vi "Multi_Run_Prog.vi"(0 "Command filename":path, 1 "Setup mode":T9(ring)) -> ()   [LabVIEW 2011]
uses:
  Anemometry Sub Vis/Gen Trav/Traverse_cluster.ctl
  Anemometry Sub Vis/Gen Trav/Spacing.ctl
  Anemometry Sub Vis/Controls/Multi_run_mode.ctl
  Anemometry Sub Vis/Gen Trav/Route mapping/Route_Display_Mode.ctl
  Anemometry Sub Vis/Controls/User_Specific_mode.ctl
  Anemometry Sub Vis/Controls/Multi_Run_Case.ctl
  Anemometry Sub Vis/Gen Trav/Multi_Run_Status.ctl
  Anemometry Sub Vis/Controls/Tunnel_Coordinates.ctl
  Anemometry Sub Vis/Controls/Post_Process.ctl
  ADAM Client/Sub VIs/ADAM Controls/Traverse_Level_State.ctl
  ADAM Client/Sub VIs/ADAM Controls/Tunnel_speed_mode.ctl
  Anemometry Sub Vis/Controls/Overhead.ctl
  ADAM Client/Sub VIs/ADAM Controls/Remember_value_mode.ctl
  Anemometry Sub Vis/Gen Trav/Trav_mode.ctl
  ADAM Client/Sub VIs/ADAM Controls/Client_Source_Status.ctl
  ADAM Client/Sub VIs/ADAM Controls/Update_scan_value.ctl
  Anemometry Sub Vis/File/Setup_Filetype.ctl
  Anemometry Sub Vis/Globals/Meas_global.vi
  Anemometry Sub Vis/Globals/Trav_pos_global.vi
  Anemometry Sub Vis/Globals/Preference_global.vi
  Anemometry Sub Vis/Gen Trav/Route mapping/Route_mapping_global.vi
  ADAM Serial/Instrument drivers/Traverses/~subVIs/DriveConfigGlobal.vi
  Anemometry Sub Vis/Globals/Extra_Commands_Global.vi
  Anemometry Sub Vis/Globals/LDA_meas_global_2.vi
  Anemometry Sub Vis/Globals/LDA_meas_global_1.vi
panel:
  out "Last Row Run":i32
  in  "Stop after Repeats":bool
  in  "Jump Bad Positions":bool
  in  "Work in Tunnel Coordinates?":T1
  out "Current Overhead Factor":dbl format="%.3f"
  out "Estimated Completion time":string
  out "Max Tunnel Speed":dbl format="%.2f"
  out "Pause message":string
  in  "Pause":bool
  out "Non Starter":bool
  out "No of Rows":i32
  out "Status":T2
  in  "Synchronization Start No":i32=1 min=1 max=100
  out "Multi Run Case":T3
  out "Simulate/Run":T4
  in  "Display Mode":T5=enum."Display View on Crash"
  in  "stop":bool
  out "Currently on Row":i32
  in  "Table":T6[](array[typedef]) {"Row Duration (mins)" format="%#.1f"; "Row No" min=0; "Trace Gas Concentration (%)" min=0.0 format="%#.2f"; "Emission Rate (l/min)" format="%#.2f"; "Tunnel Speed" format="%#.2f"; "Start X" format="%#.2f"; "Start Y" format="%#.2f"; "Start Z" format="%#.2f"; "End X" format="%#.2f"; "End Y" format="%#.2f"; "End Z" format="%#.2f"; "Averaging time (min)" min=0.0 format="%#.2f"}
  # "X           Y            Z"
  # "Start"
  # "End"
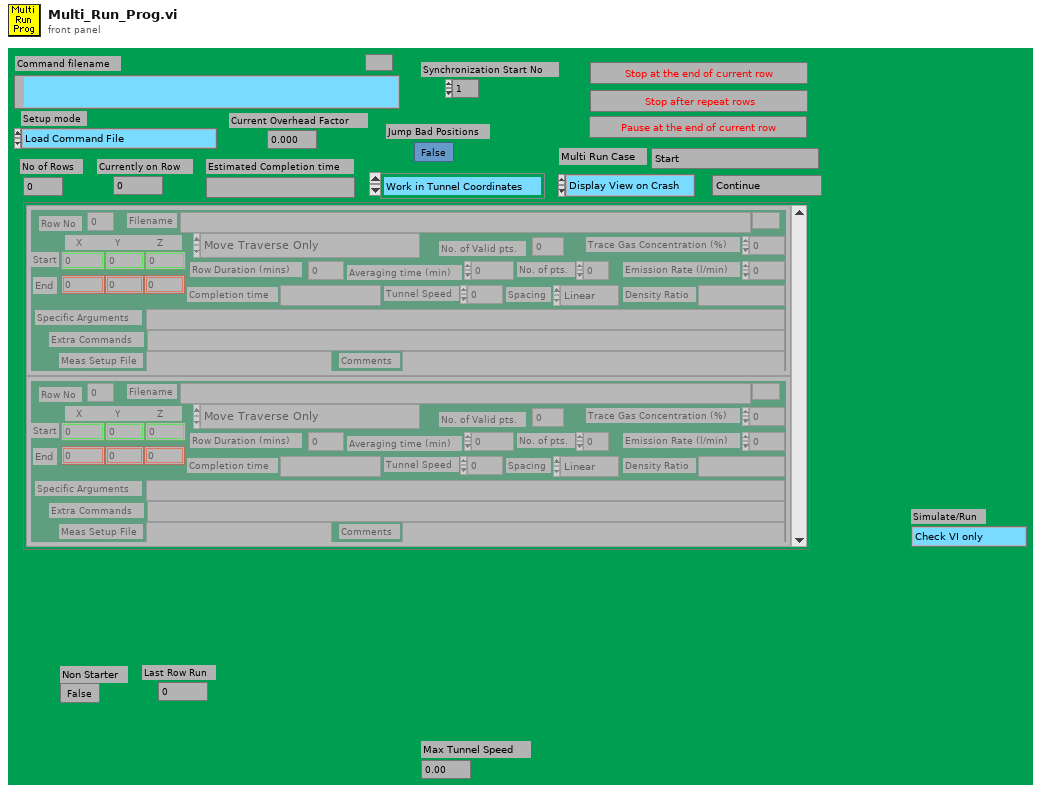
[diagram p1: front panel]
types:
  T1 = typedef "Tunnel_Coordinates.ctl" = enum16{"Work in Tunnel Coordinates", "Work in Model Coordinates"}
  T2 = typedef "Multi_Run_Status.ctl" = enum16{"Continue", "Jump to Next Point", "Jump to Next Row", "Jump To Fall Back", "Terminate Run"}
  T3 = typedef "Multi_Run_Case.ctl" = enum16{"Start", "Load Setup From File", "Has file been edited in Excel?", "Check Max Tunnel Speed", "Pre Check Row", "Check Rows", "Remove blank end rows", "Do results files already exist?", "FFID Bkgnd Measurements?", "First Save Setup file", "Setup Route checking", "Initialise Measurement Prog", "Input Current Position", "Experimental setup control", "Check source flowrates", "Setup for running mode", "Skip Blank Rows", "Which row to execute next", "Evaluate IF Statement", "Perform Measurement Setup", "Set Measurement Conditions", "Execute Row", "Calculate Row TIme", "Update time estimate", "Pause Multi Run Program", "Do Another Row?", "Find Next Fall Back Row", "Shut down source etc", "Email results to users", "Save run efficiency", "Remove Skipped Commands", "Show jumped positions", "Save Setup to File", "End"}
  T4 = typedef "User_Specific_mode.ctl" = enum16{"Check VI only", "Run VI"}
  T5 = typedef "Route_Display_Mode.ctl" = enum16{"Display View Always", "Display View on Crash"}
  T6 = typedef "Traverse_cluster.ctl" = cluster{"Start X":dbl, "Start Y":dbl, "Start Z":dbl, "End X":dbl, "End Y":dbl, "End Z":dbl, "No. of pts.":i32, "Spacing":T7, "Filename":path, "Tunnel Speed":dbl, "Averaging time (min)":dbl, "Extra Commands":string, "Specific Arguments":string, "Emission Rate (l/min)":dbl, "Trace Gas Concentration (%)":dbl, "Density Ratio":string, "Comments":string, "Row No":i32, "Row Type Selector":T8, "Completion time":string, "Row Duration (mins)":dbl, "No. of Valid pts.":i32, "Meas Setup File":string}
  T7 = typedef "Spacing.ctl" = enum16{"Linear", "Log", "Gauss", "Specified", "N/A"}
  T8 = typedef "Multi_run_mode.ctl" = enum16{"Move Traverse Only", "Set Tunnel Speed Only", "Set Source Only", "Set Measurement Conditions", "Single Measurement", "Vertical Profile", "Lateral Profile", "Longitudinal Profile", "Explore Volume", "Multi-Axis Profile", "Auto Calibrate", "Meas Fast FID Bkgnd", "Check Beam Power", "Scanning Valve Measurement", "Run VI Named:", "Set ADAM Ch", "Wait (minutes)", "Send Message", "Synchronize With:", "Fall Back to this Row", "Turn Off Row Repeating", "Blank Row"}
  T9 = enum16{"Load Command File", "Save Command File", "Check Multi Run Prog", "Check Multi Run Prog With Live Moves", "Run Multi Run Prog"}
  T10 = typedef "Post_Process.ctl" = enum16{"Take New Data", "Post Process Raw Data File"}
  T11 = typedef "Traverse_Level_State.ctl" = enum16{"Running", "Complete"}
  T12 = enum32{"existing file", "new file", "new or existing file", "existing dir", "new dir", "new or existing dir", "existing file (use LLBs)", "new file (use LLBs)", "new or existing file (use LLBs)", "new or existing file or directory (use LLBs)"}
  T13 = typedef "Tunnel_speed_mode.ctl" = enum16{"Set Speed", "Set Speed then wait", "Is tunnel speed allowable?"}
  T14 = enum16{"All Channel Names", "Valid Channel Names"}
  T15 = typedef "Overhead.ctl" = enum16{"Update total times", "Read Current Overhead", "Re Scale totals to 3 hrs", "Initialise totals to 3hr"}
  T16 = typedef "Remember_value_mode.ctl" = enum16{"Read only", "Read and Write"}
  T17 = typedef "Trav_mode.ctl" = enum16{"Move traverse", "Read traverse position", "Teach Position"}
  T18 = typedef "Client_Source_Status.ctl" = enum16{"Not Using", "Using", "Must Have"}
  T19 = typedef "Update_scan_value.ctl" = cluster{"Channel Name":string, "New Value":dbl}
  T20 = typedef "Setup_Filetype.ctl" = enum16{"Measurement Setups", "Calibration Setups", "General", "Results File Plotter Setups", "Speed Calib Tweaks"}
  T21 = typedef "AxisConfigCluster.ctl" = cluster{"Channel Properties":T22, "Static Drive Configuration":T23}
  T22 = typedef "DriveProperties.ctl" = cluster{"Channel Name":string, "Vel. Default":dbl, "Acc. Default":dbl, "Vel. Max":dbl, "Vel. Min":dbl, "Acc. Max":dbl, "Acc. Min":dbl, "Pulses/unit":dbl, "Address":u8, "Pulse Offset":i32, "Pos Tolerance":dbl, "Pulses/rev":dbl, "Backlash/Eng units":dbl, "Current Pos":dbl, "Ch Status":enum16{"Active", "Offline", "Simulate"}, "Port Name":string, "Axis Transform mode":string, "Metadata Ch Name":string, "Type":string}
  T23 = typedef "DriveStaticConfig.ctl" = cluster{"Correction Gain % (CG)":u16, "Dead Band (DB)":i32, "Dead Band Window (DW)":i32, "Encoder Resolution (ER)":i32, "Step Mode  (FSB)":u16, "Position Maintenance (FSC)":u16, "Stop on Stall (FSD)":u16, "Activate OP1 on stall (FSE)":u16, "Stop on Trigger 3 (FSF)":u16, "OP2 in Deadband (FSG)":u16, "Stall Detect (FSH)":u16, "Limit Disable (LD)":u16, "Motor Resolution (MR)":enum16{"200", "400", "1000", "2000", "4000", "5000", "10000", "12800", "18000", "20000", "21600", "25000", "25400", "25600", "36000", "50000", "278528", "425984", "507904", "614400", "655360", "819200", "1024000"}, "Limit Switch Sense (OSA)":u16, "Home Position (OSB)":u16, "Home Switch Sense (OSC)":u16, "Encoder Z for Home (OSD)":u16, "Reference edge of Home (OSH)":u16, "RS232 Echo Control (SSA)":u16, "Buffer at Limit (SSG)":u16, "Buffer at Stop (SSH)":u16, "Indexer Mode  (FSA)":u16, "Type":string, "ConfigString":string, "De Power Motor":enum16{"TRUE", "FALSE"}}
  T24 = typedef "Status_Cluster.ctl" = cluster{"Status":T2, "Error Type":string, "Error Description":string}
  T25 = typedef "BSA_info_Cluster.ctl" = cluster{"GPIB Address":string, "No of Check Bytes":i32, "Extra Info":string, "COLOUR":u32, "Wavelength (nm)":dbl}
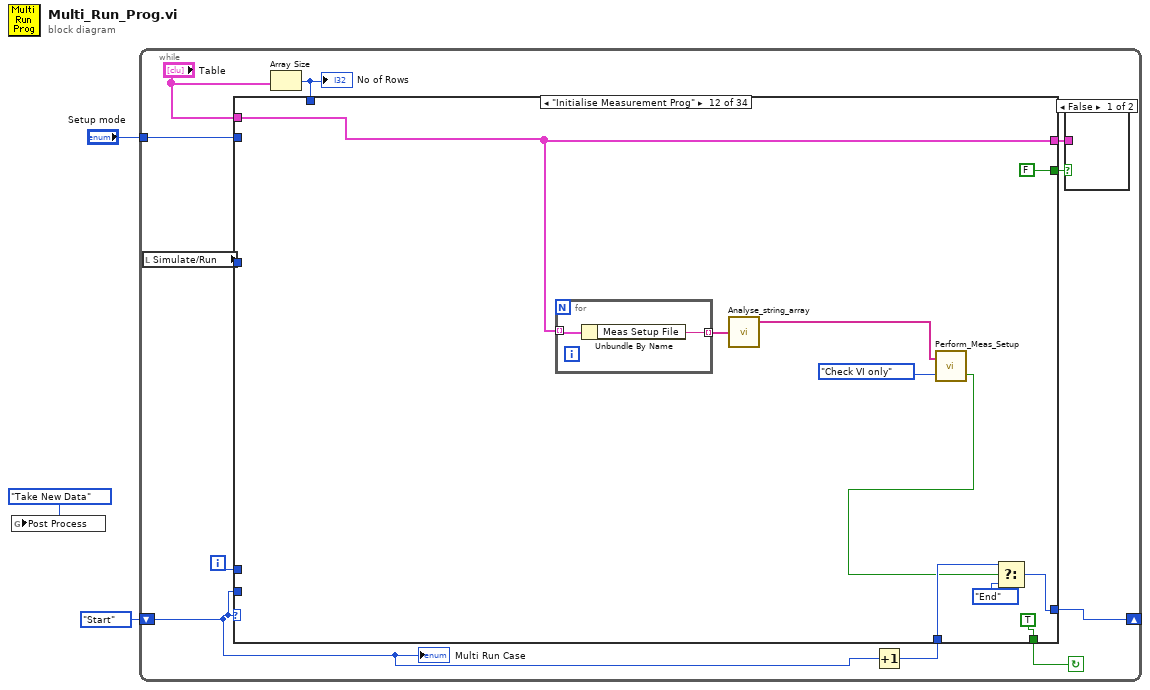
[diagram p0: block diagram]
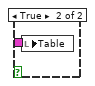
[diagram p2: hidden frame]
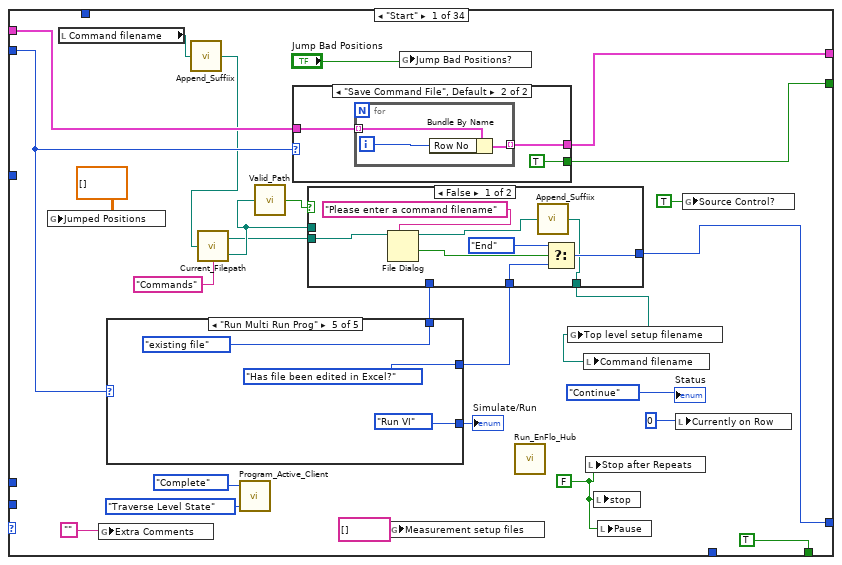
[diagram p3: hidden frame]
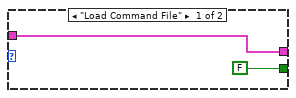
[diagram p4: hidden frame]
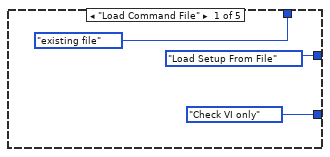
[diagram p6: hidden frame]
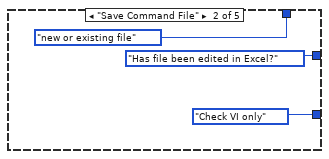
[diagram p7: hidden frame]
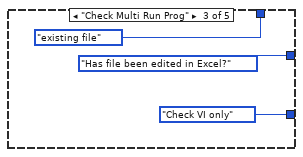
[diagram p8: hidden frame]
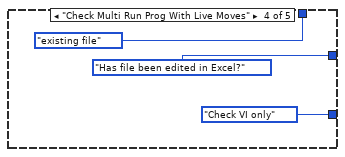
[diagram p9: hidden frame]
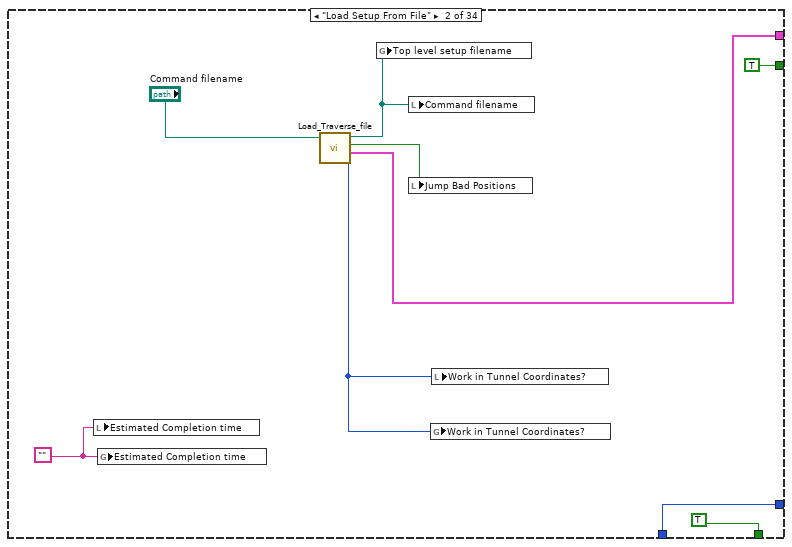
[diagram p10: hidden frame]
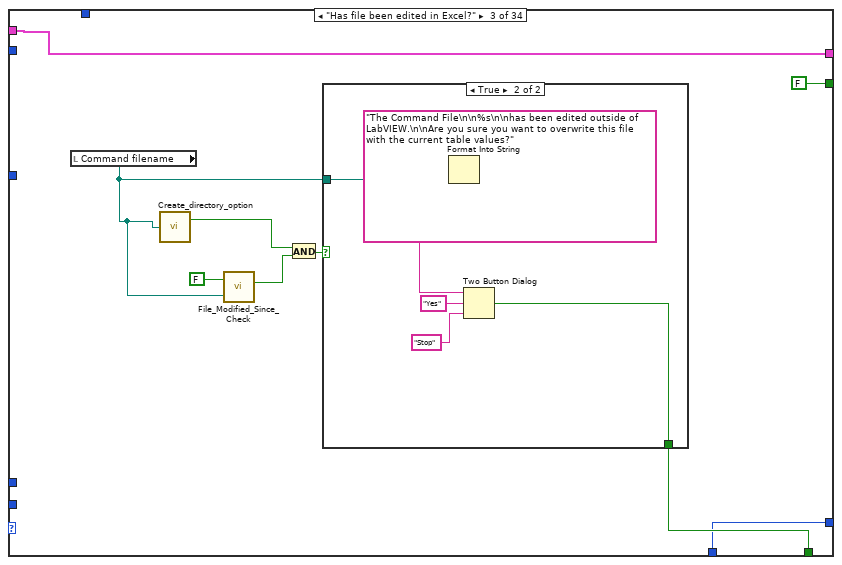
[diagram p11: hidden frame]
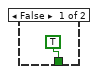
[diagram p12: hidden frame]
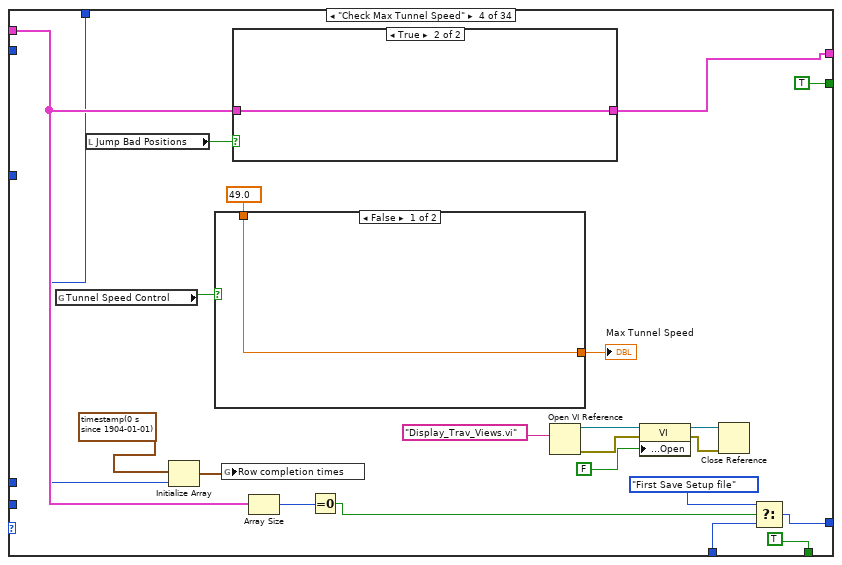
[diagram p13: hidden frame]
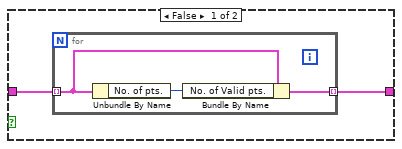
[diagram p14: hidden frame]
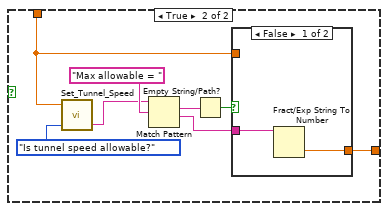
[diagram p15: hidden frame]
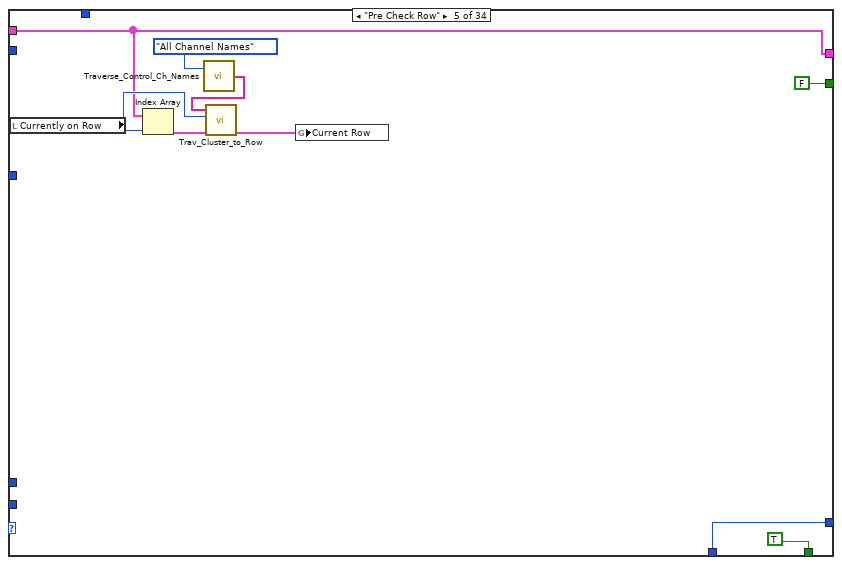
[diagram p17: hidden frame]
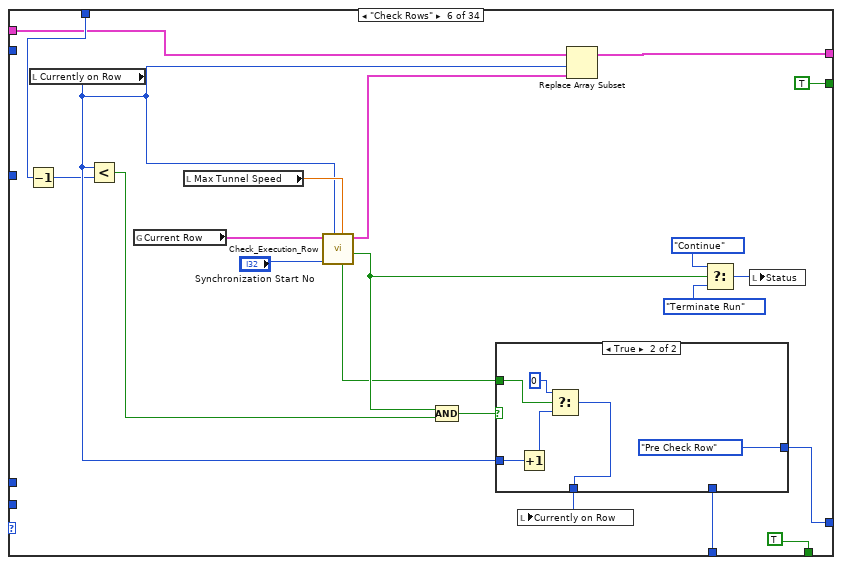
[diagram p18: hidden frame]
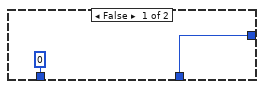
[diagram p19: hidden frame]
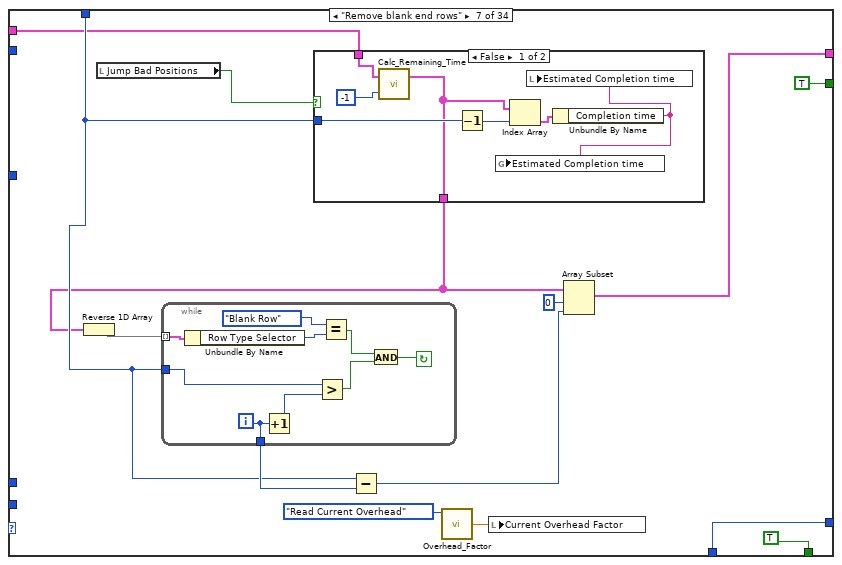
[diagram p20: hidden frame]
diagram:
  n1 = global write "Meas_global.vi" "Post Process"(Post_Process."Take New Data" ("Post Process")) -> ()
  n2 = while {
    shift-left: Multi_Run_Case."Start" ("Multi Run Case") -> [w10]
    shift-right: [w6] -> _
    tunnel: "Setup mode" -> [w13]
    i -> [w11]
    stop <- w14 continue-if-true
    n3 = local read "Simulate/Run"() -> (w7:T4)
    n4 = Array Size(array="Table") -> (size(s)=w5:i32)
    "No of Rows" <- w5
    n5 = Increment(x=w10) -> (x+1=w12:T3)
    n6 = case shown="\"Initialise Measurement Prog\"" w10 {
      tunnel: [TRUE TRUE w87 TRUE TRUE TRUE TRUE TRUE TRUE TRUE TRUE ("Continue?") TRUE ("Continue?") TRUE TRUE TRUE w506 TRUE ("Continue?") TRUE ("Continue?") TRUE TRUE ("Continue?") TRUE TRUE TRUE TRUE TRUE TRUE TRUE TRUE TRUE TRUE TRUE TRUE TRUE FALSE] -> w14
      tunnel: w13 -> [w26 _ _ _ _ _ _ _ _ w395 _ _ _ _ _ _ _ _ _ _ _ _ _ _ _ _ _ _ _ _ _ _ w1220 _]
      tunnel: "Table" -> [w39 _ w84 w114 w142 w154 w179 w210 w368 w397 w419 w472 w477 w483 w493 w509 w561 w605 w721 w772 w784 w875 w911 w943 w984 w1026 w1061 w1091 w1120 w1165 w1170 w1179 w1241 w1304]
      tunnel: w7 -> [_ _ _ _ _ _ _ w209 _ _ _ _ _ w487 w492 w508 _ w603 w718 w769 w782 w874 w909 w940 _ w1035 _ w1082 _ _ _ _ w1231 _]
      tunnel: w10 -> [_ _ _ _ _ _ _ _ _ _ _ _ _ _ _ _ _ _ _ _ _ _ _ _ _ _ _ _ _ _ _ _ _ _]
      tunnel: w12 -> [_ w80 w86 w112 w146 w156 w190 w214 w363 w394 w423 w470 w478 w482 w498 w511 w563 w601 w726 w773 w791 w872 w901 w945 w987 _ _ w1075 w1122 w1167 w1173 w1187 w1239 w1303]
      tunnel: w11 -> [_ _ _ _ _ _ _ _ _ _ _ _ _ _ _ _ _ _ _ _ _ _ _ _ w985 _ _ _ _ _ _ _ _ _]
      tunnel: [w37 w80 w86 w111 w146 w155 w190 w214 w363 w390 w423 w469 w478 w482 w495 w511 w563 w602 w725 w773 w792 w872 w901 w945 w988 w1036 w1058 w1086 w1122 w1167 w1173 w1187 w1239 w1303] -> w6
      tunnel: [w25 TRUE FALSE ("Rows Added ?") TRUE ("Rows Added ?") FALSE TRUE TRUE FALSE FALSE TRUE FALSE FALSE FALSE FALSE FALSE TRUE FALSE ("Rows Added ?") FALSE ("Rows Added ?") FALSE FALSE ("Rows Added ?") FALSE FALSE FALSE TRUE ("Rows Added ?") FALSE FALSE FALSE FALSE FALSE FALSE TRUE TRUE TRUE FALSE] -> w8
      tunnel: w5 -> [_ _ _ w106 _ w160 w181 _ _ _ _ _ _ _ _ _ w564 w604 _ _ _ _ _ w939 _ w1021 _ _ _ _ _ _ _ _]
      tunnel: [w38 w81 w84 w116 w142 w163 w185 w210 w368 w398 w419 w472 w477 w483 w493 w507 w561 w606 w721 w772 w784 w875 w911 w942 w984 w1026 w1061 w1091 w1120 w1165 w1169 w1179 w1240 w1304] -> w4
      frame "Start" {
        w23 = FALSE ("Measurment setup Found?")
        n7 = global write "Trav_pos_global.vi" "Jumped Positions"(dbl[][] [] ("Jumped Positions")) -> ()
        n8 = local read "Command filename"() -> (w29:path)
        n9 = global write "Meas_global.vi" "Extra Comments"("") -> ()
        n10 = case shown="\"Run Multi Run Prog\"" w26 {
          tunnel: [User_Specific_mode."Check VI only" ("Simulate/Run") User_Specific_mode."Check VI only" ("Simulate/Run") User_Specific_mode."Check VI only" ("Simulate/Run") User_Specific_mode."Check VI only" ("Simulate/Run") User_Specific_mode."Run VI" ("Simulate/Run")] -> w40
          tunnel: [Multi_Run_Case."Load Setup From File" ("Multi Run Case") Multi_Run_Case."Has file been edited in Excel?" ("Multi Run Case") Multi_Run_Case."Has file been edited in Excel?" ("Multi Run Case") Multi_Run_Case."Has file been edited in Excel?" ("Multi Run Case") Multi_Run_Case."Has file been edited in Excel?" ("Multi Run Case")] -> w36
          tunnel: [T12."existing file" ("select mode (2)") T12."new or existing file" ("select mode (2)") T12."existing file" ("select mode (2)") T12."existing file" ("select mode (2)") T12."existing file" ("select mode (2)")] -> w24
          frame "Load Command File" {
          }
          frame "Save Command File" {
          }
          frame "Check Multi Run Prog" {
          }
          frame "Check Multi Run Prog With Live Moves" {
          }
          frame "Run Multi Run Prog" {
          }
        }
        "Simulate/Run" <- w40
        n11 = call "Append_Suffiix.vi"("Results file"=w29) -> ("appended path"=w18:path)
        n12 = call "Current_Filepath.vi"("Filename in"=w18, "Data Type"="Commands") -> ("Filename Out"=w17:path, "Directory"=w16:path)
        n13 = call "Program_Active_Client.vi"("Mode"=enum16{"Program Active", "Traverse Level State"}."Traverse Level State", "Traverse level State"=Traverse_Level_State."Complete") -> ()  [unwired: 1 in, 3 out]
        n14 = call "Valid_Path.vi"("Filename"=w17) -> ("Valid Path?"=w27:bool)
        n15 = case shown="\"Save Command File\", Default" w26 {
          tunnel: w39 -> [w43 w46]
          tunnel: [w43 w45] -> w38
          tunnel: [FALSE TRUE] -> w25
          frame "Load Command File" {
          }
          frame "Save Command File", Default {
            n16 = for {
              tunnel: w46 -> [w49] mode=indexing
              tunnel: [w48] -> w45 mode=indexing
              i -> [w47]
              n17 = Bundle By Name(cluster=w49, "Row No"=w47) -> (w48:T6)
            }
          }
        }
        n18 = case shown="False" w27 {
          tunnel: [w55 w59] -> w37
          tunnel: w36 -> [w56 w59]
          tunnel: w17 -> [_ w58]
          tunnel: [w54 w58] -> w28
          tunnel: w24 -> [_ _]
          tunnel: w16 -> [w50 _]
          frame False {
            n19 = File Dialog(7:"Please enter a command filename" ("prompt"), 11:w50) -> (1:w52:bool, 3:w53:path)  [unwired: 1 in, 6 out]
            n20 = call "Append_Suffiix.vi"("Results file"=w53) -> ("appended path"=w54:path)
            n21 = Select(t=Multi_Run_Case."End" ("Multi Run Case"), s=w52, f=w56) -> (s? t:f=w55:T3)
          }
          frame True {
          }
        }
        n22 = global write "Trav_pos_global.vi" "Measurement setup files"(string[] [] ("Measurement setup files")) -> ()
        n23 = global write "Trav_pos_global.vi" "Jump Bad Positions?"("Jump Bad Positions") -> ()
        n24 = call "Run_EnFlo_Hub.vi"() -> ()  [unwired: 8 out]
        n25 = global write "Trav_pos_global.vi" "Top level setup filename"(w28) -> ()
        n26 = local write "Command filename"(w28) -> ()
        n27 = local write "Stop after Repeats"(w23) -> ()
        n28 = local write "stop"(w23) -> ()
        n29 = local write "Pause"(w23) -> ()
        n30 = local write "Currently on Row"(0 ("Currently on Row")) -> ()
        n31 = global write "Trav_pos_global.vi" "Source Control?"(TRUE ("Source Control?")) -> ()
        "Status" <- Multi_Run_Status."Continue" ("Status")
      }
      frame "Load Setup From File" {
        w76 = ""
        n32 = local write "Estimated Completion time"(w76) -> ()
        n33 = global write "Trav_pos_global.vi" "Estimated Completion time"(w76) -> ()
        n34 = call "Load_Traverse_file.vi"("Setup filename"="Command filename") -> ("Setup filename Out"=w78:path, "Jump Bad Positions"=w75:bool, "Table"=w81:T6[], "Work in Tunnel Coordinates?"=w77:T1)  [unwired: 2 out]
        n35 = global write "Trav_pos_global.vi" "Top level setup filename"(w78) -> ()
        n36 = local write "Command filename"(w78) -> ()
        n37 = local write "Jump Bad Positions"(w75) -> ()
        n38 = global write "Trav_pos_global.vi" "Work in Tunnel Coordinates?"(w77) -> ()
        n39 = local write "Work in Tunnel Coordinates?"(w77) -> ()
      }
      frame "Has file been edited in Excel?" {
        n40 = local read "Command filename"() -> (w88:path)
        n41 = call "Create_directory_option.vi"("Filename"=w88) -> ("Path is to existing File"=w91:bool)  [unwired: 1 out]
        n42 = call "File_Modified_Since_Check.vi"("Pathname"=w88, "Just Modified?"=FALSE) -> ("Modified?"=w90:bool)
        n43 = And(x=w91, y=w90) -> (x .and. y?=w92:bool)
        n44 = case shown="True" w92 {
          tunnel: w88 -> [_ w99]
          tunnel: [TRUE ("T button?") w94] -> w87
          frame False {
          }
          frame True {
            n45 = Format Into String(format string="The Command File\n\n%s\n\nhas been edited outside of LabVIEW.\n\nAre you sure you want to overwrite this file  with the current table values?" ("Format String"), w99) -> (resulting string=w97:string)  [unwired: 2 in, 1 out]
            n46 = Two Button Dialog(message=w97, 1:"Stop" ("F button name (\"Cancel\")"), 2:"Yes" ("T button name (\"OK\")")) -> (T button?=w94:bool)
          }
        }
      }
      frame "Check Max Tunnel Speed" {
        n47 = global read "Preference_global.vi" "Tunnel Speed Control"() -> (w117:bool)
        n48 = local read "Jump Bad Positions"() -> (w115:bool)
        n49 = Initialize Array(timestamp(0 s since 1904-01-01) ("seconds since 1Jan1904"), w106) -> (w107:timestamp[])
        n50 = case shown="False" w117 {
          tunnel: 49.0 ("Tunnel Velocity m/s") -> [w128 w129]
          tunnel: [w128 w131] -> w119
          frame False {
          }
          frame True {
            n51 = call "Set_Tunnel_Speed.vi"("Mode"=Tunnel_speed_mode."Is tunnel speed allowable?", "Tunnel Velocity m/s"=w129) -> ("Error String"=w134:string)  [unwired: 1 in, 2 out]
            n52 = Match Pattern(string=w134, regular expression="Max allowable = ") -> (match substring=w133:string, after substring=w130:string)  [unwired: 3 out]
            n53 = Empty String/Path?(string/path=w133) -> (empty?=w132:bool)
            n54 = case shown="False" w132 {
              tunnel: [w137 w139] -> w131
              tunnel: w129 -> [_ w139]
              tunnel: w130 -> [w138 _]
              frame False {
                n55 = Fract/Exp String To Number(string=w138) -> (number=w137:dbl)  [unwired: 4 out]
              }
              frame True {
              }
            }
          }
        }
        "Max Tunnel Speed" <- w119
        n56 = global write "Trav_pos_global.vi" "Row completion times"(w107) -> ()
        n57 = case shown="True" w115 {
          tunnel: w114 -> [w123 w127]
          tunnel: [w122 w127] -> w116
          frame False {
            n58 = for {
              tunnel: w123 -> [w125] mode=indexing
              tunnel: [w124] -> w122 mode=indexing
              n59 = Unbundle By Name(w125) -> ("No. of pts."=w126:i32)
              n60 = Bundle By Name(cluster=w125, "No. of Valid pts."=w126) -> (w124:T6)
            }
          }
          frame True {
          }
        }
        n61 = Array Size(array=w114) -> (size(s)=w113:i32)
        n62 = Equal To 0?(x=w113) -> (x = 0?=w110:bool)
        n63 = Open VI Reference(vi path="Display_Trav_Views.vi" ("VI path")) -> (vi reference=w105:refnum<vi>, error out=w104:errorcluster)  [unwired: 1 in, 4 out]
        n64 = property class="VI"(reference=w105, error in=w104, "Front Panel Window:Open"=FALSE) -> (reference out=w102:refnum<vi>, error out=w101:errorcluster)
        n65 = Close Reference(reference=w102, error in (no error)=w101) -> ()  [unwired: 1 out]
        n66 = Select(t=Multi_Run_Case."First Save Setup file" ("Multi Run Case"), s=w110, f=w112) -> (s? t:f=w111:T3)
      }
      frame "Pre Check Row" {
        n67 = local read "Currently on Row"() -> (w143:i32)
        n68 = Index Array(array=w142, index=w143) -> (element=w144:T6)
        n69 = call "Traverse_Control_Ch_Names.vi"("Mode"=T14."All Channel Names") -> ("Channel names"=w140:string[])  [unwired: 1 in]
        n70 = call "Trav_Cluster_to_Row.vi"("Traverse line in"=w144, "Row Number"=w143, "Channel names"=w140) -> ("Traverse line Out"=w145:T6)  [unwired: 4 out]
        n71 = global write "Trav_pos_global.vi" "Current Row"(w145) -> ()
      }
      frame "Check Rows" {
        n72 = Decrement(x=w160) -> (x-1=w150:i32)
        n73 = local read "Currently on Row"() -> (w151:i32)
        n74 = Less?(x=w151, y=w150) -> (x < y?=w159:bool)
        n75 = global read "Trav_pos_global.vi" "Current Row"() -> (w152:T6)
        n76 = local read "Max Tunnel Speed"() -> (w162:dbl)
        n77 = call "Check_Execution_Row.vi"("Execution Row"=w152, "Synchronization Start No"="Synchronization Start No", "Row Index"=w151, "Max Tunnel Speed"=w162) -> ("Editted Row"=w149:bool, "Execution Row Out"=w153:T6, "Continue?"=w161:bool)  [unwired: 1 in, 3 out]
        n78 = Compound Arithmetic op=AND(w161, w159) -> (w158:bool)
        n79 = case shown="True" w158 {
          tunnel: [0 w173] -> w157
          tunnel: w151 -> [_ w177]
          tunnel: w156 -> [w171 _]
          tunnel: [w171 Multi_Run_Case."Pre Check Row" ("Multi Run Case")] -> w155
          tunnel: w149 -> [_ w175]
          frame False {
          }
          frame True {
            n80 = Increment(x=w177) -> (x+1=w174:i32)
            n81 = Select(t=0, s=w175, f=w174) -> (s? t:f=w173:i32)
          }
        }
        n82 = local write "Currently on Row"(w157) -> ()
        n83 = Replace Array Subset(array=w154, new element=w153, index=w151) -> (w163:T6[])
        n84 = Select(t=Multi_Run_Status."Continue" ("Status"), s=w161, f=Multi_Run_Status."Terminate Run" ("Status")) -> (s? t:f=w167:T2)
        n85 = local write "Status"(w167) -> ()
      }
      frame "Remove blank end rows" {
        n86 = local read "Jump Bad Positions"() -> (w178:bool)
        n87 = case shown="False" w178 {
          tunnel: w181 -> [w196 _]
          tunnel: w179 -> [w195 w199]
          tunnel: [w193 w199] -> w180
          frame False {
            n88 = call "Calc_Remaining_Time.vi"("Currently on Row"=-1 ("Start Index"), "Table In"=w195) -> ("Table Out"=w193:T6[])  [unwired: 1 out]
            n89 = Decrement(x=w196) -> (x-1=w198:i32)
            n90 = Index Array(array=w193, index=w198) -> (element=w197:T6)
            n91 = Unbundle By Name(w197) -> ("Completion time"=w192:string)
            n92 = global write "Trav_pos_global.vi" "Estimated Completion time"(w192) -> ()
            n93 = local write "Estimated Completion time"(w192) -> ()
          }
          frame True {
          }
        }
        n94 = Reverse 1D Array(array=w180) -> (reversed array=w189:T6[])
        n95 = while {
          tunnel: [w200] -> w187
          tunnel: w181 -> [w204]
          tunnel: w189 -> [w208] mode=indexing
          i -> [w200]
          stop <- w201 continue-if-true
          n96 = Unbundle By Name(w208) -> ("Row Type Selector"=w206:T8)
          n97 = Increment(x=w200) -> (x+1=w205:i32)
          n98 = Greater?(x=w204, y=w205) -> (0:w203:bool)
          n99 = Equal?(x=Multi_run_mode."Blank Row" ("Row Type Selector"), y=w206) -> (x = y?=w202:bool)
          n100 = And(x=w202, y=w203) -> (x .and. y?=w201:bool)
        }
        n101 = Subtract(x=w181, y=w187) -> (x-y=w186:i32)
        n102 = call "Overhead_Factor.vi"("Mode"=Overhead."Read Current Overhead") -> ("Current Overhead Factor"=w182:dbl)  [unwired: 3 in]
        n103 = local write "Current Overhead Factor"(w182) -> ()
        n104 = Array Subset(array=w180, index=0 ("Array Index"), length=w186) -> (w185:T6[])
      }
      frame "Do results files already exist?" {
        n105 = for {
          tunnel: w210 -> [w226] mode=indexing
          tunnel: [w224] -> w216 mode=indexing
          shift-right: [w220] -> _
          shift-left: path[] [] -> [w221]
          tunnel: w209 -> [w218]
          n106 = Unbundle By Name(w226) -> ("Specific Arguments"=w217:string, "Emission Rate (l/min)"=w225:dbl, "Row Type Selector"=w223:T8, "Filename"=w222:path)
          n107 = while {
            shift-left: w221 -> [w234]
            shift-right: [w233] -> w220
            tunnel: w222 -> [w235]
            tunnel: w223 -> [w239]
            shift-left: 0 -> [w240]
            shift-right: [w236] -> _
            tunnel: w218 -> [w230]
            shift-right: [w229] -> _
            shift-left: _ -> [w228]
            tunnel: w217 -> [w227]
            stop <- w238 continue-if-true
            n108 = Increment(x=w240) -> (x+1=w237:i32)
            n109 = case shown="0, Default" w240 {
              tunnel: w239 -> [w249 _ _ _ _ _ _ _ _ _ _ _]
              tunnel: [w244 w269 w274 w281 w286 TRUE ("exists?") TRUE ("exists?") FALSE ("exists?") FALSE ("exists?") TRUE ("true") w343 w356] -> w238
              tunnel: w237 -> [w251 w272 w277 w280 w287 w292 w303 w314 w325 w329 w341 _]
              tunnel: [w251 w272 w277 w280 w287 w290 w302 w314 w325 w330 w341 w355] -> w236
              tunnel: [w250 w271 w276 w279 w284 w300 w311 w316 w318 w327 w345 w361] -> w233
              tunnel: w234 -> [w250 w271 w276 w279 w285 w300 w311 w316 w318 w327 w345 w361]
              tunnel: w235 -> [w243 _ _ _ _ _ _ _ _ _ _ _]
              tunnel: 7 -> [_ _ _ _ _ _ _ _ _ w328 _ w355]
              tunnel: 9 -> [_ _ _ _ _ w291 _ _ _ _ _ _]
              tunnel: w230 -> [_ _ _ _ _ _ _ _ _ _ w344 _]
              tunnel: [w242 w268 w273 w278 w283 w288 w301 w312 w317 w326 w342 w354] -> w229
              tunnel: w228 -> [_ w268 w273 w278 w283 w288 w301 w312 w317 w326 w342 w354]
              tunnel: w227 -> [w241 _ _ _ _ _ _ _ _ _ _ _]
              frame 0, Default {
                n110 = case shown="\"Run VI Named:\"" w249 {
                  tunnel: [TRUE w259 FALSE FALSE] -> w246
                  tunnel: w243 -> [w252 w258 w264 w266]
                  tunnel: w241 -> [_ w256 _ _]
                  tunnel: [w252 w258 w264 w266] -> w242
                  frame "Move Traverse Only", Default {
                  }
                  frame "Run VI Named:" {
                    n111 = Match Pattern(string=w256, regular expression=";") -> (before substring=w255:string)  [unwired: 4 out]
                    n112 = call <vilib>:"Trim Whitespace.vi"("string"=w255) -> ("trimmed string"=w254:string)  [unwired: 1 in]
                    n113 = Equal?(x=w254, y="Pressure_Tapped_Cube.vi") -> (x = y?=w260:bool)
                    n114 = Equal?(x=w254, y="Take_Data_on_the_Move.vi") -> (x = y?=w261:bool)
                    n115 = Or(x=w260, y=w261) -> (x .or. y?=w259:bool)
                  }
                  frame "Auto Calibrate" {
                  }
                  frame "Send Message" {
                  }
                }
                n116 = local read "Status"() -> (w247:T2)
                n117 = Not Equal?(x=Multi_Run_Status."Terminate Run" ("Status"), y=w247) -> (x != y?=w245:bool)
                n118 = And(x=w246, y=w245) -> (x .and. y?=w244:bool)
              }
              frame 1 {
                n119 = Not Equal?(x=path "", y=w268) -> (x != y?=w269:bool)
              }
              frame 2 {
                n120 = Not Equal?(x=w273, y=path "") -> (x != y?=w274:bool)
              }
              frame 3 {
                n121 = Search 1D Array(1D array=w279, element=w278) -> (index of element=w282:i32)  [unwired: 1 out]
                n122 = Less Than 0?(x=w282) -> (x < 0?=w281:bool)
              }
              frame 4 {
                n123 = Build Array (concatenate)(w285, w283) -> (w284:path[])
                n124 = call "Does_file_exist_(simple).vi"("Pathname"=w283) -> ("exists?"=w286:bool)
              }
              frame 5 {
                n125 = Path To String(path=w288) -> (string=w299:string)
                n126 = global read "Meas_global.vi" "Start Time of experiment"() -> (w294:dbl)
                n127 = Concatenate Strings(w299, "Append" ("Substring")) -> (w297:string)
                n128 = call "Remember_value.vi"("Mode"=Remember_value_mode."Read only", "Ch name"=w297) -> ("Output Value"=w295:dbl)  [unwired: 1 in]
                n129 = Not Equal?(x=w294, y=w295) -> (x != y?=w293:bool)
                n130 = Select(t=w292, s=w293, f=w291) -> (s? t:f=w290:i32)
              }
              frame 6 {
                n131 = Increment(x=w303) -> (x+1=w304:i32)
                n132 = Format Into String(format string="The results filename \"%s\" already exists.\nDo you wish to append to this file during the run?" ("Format String"), w301) -> (resulting string=w308:string)  [unwired: 2 in, 1 out]
                n133 = Two Button Dialog(message=w308, 1:"Abort Run" ("F button name (\"Cancel\")"), 2:"Append" ("T button name (\"OK\")")) -> (T button?=w305:bool)
                n134 = Select(t=w304, s=w305, f=w303) -> (s? t:f=w302:i32)
              }
              frame 7 {
                n135 = local write "Status"(Multi_Run_Status."Terminate Run" ("Status")) -> ()
              }
              frame 8 {
                n136 = Path To String(path=w317) -> (string=w324:string)
                n137 = Concatenate Strings(w324, "Append" ("Substring")) -> (w322:string)
                n138 = global read "Meas_global.vi" "Start Time of experiment"() -> (w319:dbl)
                n139 = call "Remember_value.vi"("Mode"=Remember_value_mode."Read and Write", "Input Value"=w319, "Ch name"=w322) -> ()  [unwired: 1 out]
              }
              frame 9 {
                n140 = call "Read_File_Simple.vi"("Filename"=w326) -> ("string"=w333:string)  [unwired: 2 in, 7 out]
                n141 = call "Is_it_a_Results_File.vi"("character string"=w333) -> ("Results File?"=w332:bool)  [unwired: 2 out]
                n142 = case shown="True" w332 {
                  tunnel: w326 -> [w336 _]
                  tunnel: [w334 w340] -> w330
                  tunnel: w329 -> [_ w340]
                  tunnel: w328 -> [w334 _]
                  frame False {
                    n143 = Path To String(path=w336) -> (string=w338:string)
                    n144 = Format Into String(format string="The File %s is not in the correct Results file format.\nCheck that it is tab delimited rather than excel format, or choose another file." ("Format String"), w338) -> (resulting string=w335:string)  [unwired: 2 in, 1 out]
                    n145 = One Button Dialog(message=w335, button name ("OK")="Stop") -> ()  [unwired: 1 out]
                  }
                  frame True {
                  }
                }
              }
              frame 10 {
                n146 = case shown="\"Check VI only\", Default" w344 {
                  tunnel: w342 -> [_ w353]
                  tunnel: [FALSE ("exists?") w347] -> w343
                  frame "Check VI only", Default {
                  }
                  frame "Run VI" {
                    n147 = call "Open_File_for_write.vi"("append to file? (new file:F)"=TRUE, "file path"=w353) -> ("error out"=w351:errorcluster, "refnum"=w352:refnum<file>)  [unwired: 1 in, 7 out]
                    n148 = Unbundle By Name(w351) -> ("code"=w350:i32)
                    n149 = Close File(refnum=w352, error in=w351) -> ()  [unwired: 2 out]
                    n150 = Equal?(x=10 ("code"), y=w350) -> (x = y?=w347:bool)
                  }
                }
              }
              frame 11 {
                n151 = Path To String(path=w354) -> (string=w359:string)
                n152 = Format Into String(format string="The File %s is already open in another application." ("Format String"), w359) -> (resulting string=w358:string)  [unwired: 2 in, 1 out]
                n153 = One Button Dialog(message=w358, button name ("OK")="Stop") -> (true=w356:bool)
              }
            }
          }
          n154 = Greater Than 0?(x=w225) -> (x > 0?=w224:bool)
        }
        n155 = Or Array Elements(Boolean array=w216) -> (logical OR=w212:bool)
        n156 = global write "Trav_pos_global.vi" "Source Control?"(w212) -> ()
      }
      frame "FFID Bkgnd Measurements?" {
        n157 = for {
          tunnel: w368 -> [w384] mode=indexing
          tunnel: [w372] -> w367 mode=indexing
          tunnel: [w373] -> w366 mode=indexing
          n158 = Unbundle By Name(w384) -> ("Row Type Selector"=w378:T8, "Specific Arguments"=w380:string)
          n159 = call "Get_array_values_fr_String.vi"("String Value"=w380) -> ("String array"=w381:string[])  [unwired: 1 out]
          n160 = Index Array(array=w381, index=0 ("Index")) -> (element=w377:string)
          n161 = Equal?(x=Multi_run_mode."Auto Calibrate" ("Row Type Selector"), y=w378) -> (x = y?=w374:bool)
          n162 = Equal?(x=w377, y="Concentration") -> (x = y?=w375:bool)
          n163 = Equal?(x=Multi_run_mode."Meas Fast FID Bkgnd" ("Row Type Selector"), y=w378) -> (x = y?=w372:bool)
          n164 = And(x=w374, y=w375) -> (x .and. y?=w373:bool)
        }
        n165 = Or Array Elements(Boolean array=w367) -> (logical OR=w364:bool)
        n166 = Or Array Elements(Boolean array=w366) -> (logical OR=w365:bool)
        n167 = Compound Arithmetic op=AND(invert w364, w365) -> (w362:bool)
        n168 = case shown="True" w362 {
          frame False {
          }
          frame True {
            n169 = One Button Dialog(message="This run automatically calibrates the Fast FID but does not have a Meas Fast FID Bkgnd row" ("format string")) -> ()  [unwired: 2 out]
          }
        }
      }
      frame "First Save Setup file" {
        w385 = -1 ("Currently on Row")
        n170 = case shown="\"Check Multi Run Prog\"" w395 {
          tunnel: [w402 w404 w406 Multi_Run_Case."End" ("Multi Run Case") Multi_Run_Case."End" ("Multi Run Case")] -> w389
          tunnel: w394 -> [w402 w404 w406 _ _]
          tunnel: [w403 w405 w407 w408 w410] -> w388
          frame "Run Multi Run Prog" {
            w403 = FALSE  # Live Traverse Preview?
          }
          frame "Check Multi Run Prog With Live Moves" {
            w405 = TRUE  # Live Traverse Preview?
          }
          frame "Check Multi Run Prog" {
            w407 = FALSE  # Live Traverse Preview?
          }
          frame "Load Command File" {
            w408 = FALSE  # Live Traverse Preview?
          }
          frame "Save Command File" {
            w410 = FALSE  # Live Traverse Preview?
          }
        }
        n171 = local read "Command filename"() -> (w396:path)
        n172 = global write "Trav_pos_global.vi" "Work in Tunnel Coordinates?"("Work in Tunnel Coordinates?") -> ()
        n173 = local write "Currently on Row"(w385) -> ()
        n174 = local write "Last Row Run"(w385) -> ()
        n175 = local read "Jump Bad Positions"() -> (w386:bool)
        n176 = call "Save_Trav_setup.vi"("Work in Tunnel Coordinates?"="Work in Tunnel Coordinates?", "Trav Table"=w397, "Jump Bad Positions"=w386, "Setup filename"=w396) -> ("Trav Table Out"=w398:T6[])  [unwired: 1 out]
        n177 = global write "Meas_global.vi" "Extra Comments"("") -> ()
        n178 = global write "Trav_pos_global.vi" "Live Traverse Preview?"(w388) -> ()
        n179 = local read "Status"() -> (w391:T2)
        n180 = case shown="\"Continue\"" w391 {
          tunnel: [w400 Multi_Run_Case."End" ("Multi Run Case")] -> w390
          tunnel: w389 -> [w400 _]
          frame "Continue" {
          }
          frame "Jump to Next Point", Default {
          }
        }
      }
      frame "Setup Route checking" {
        w414 = string[] []
        n181 = global read "Trav_pos_global.vi" "Work in Tunnel Coordinates?"() -> (w416:T1)
        n182 = for {
          tunnel: w419 -> [w459] mode=indexing
          shift-right: [w450] -> w417
          shift-left: string[] [] -> [w451]
          n183 = Unbundle By Name(w459) -> ("Extra Commands"=w452:string, "Start X"=w456:dbl, "Start Y"=w455:dbl, "Start Z"=w454:dbl)
          n184 = Build Array(w456, w455, w454) -> (w457:dbl[])
          n185 = Not A Number/Path/Refnum?(number/path/refnum=w457) -> (NaN/Path/Refnum?=w458:bool[])
          n186 = Or Array Elements(Boolean array=w458) -> (logical OR=w453:bool)
          n187 = case shown="False" w453 {
            tunnel: w452 -> [w463 _]
            tunnel: w451 -> [w462 w464]
            tunnel: [w461 w464] -> w450
            frame False {
              n188 = call "Which_Trav_Setup.vi"("Extra Command String"=w463) -> ("Traverse Setup"=w460:string)
              n189 = Build Array (concatenate)(w462, w460) -> (w461:string[])
            }
            frame True {
            }
          }
        }
        n190 = call "Analyse_string_array.vi"("String array"=w417) -> ("Unique strings"=w415:string[])  [unwired: 2 out]
        n191 = for {
          tunnel: w415 -> [w429] mode=indexing
          tunnel: w416 -> [w428]
          shift-right: [w427] -> w412
          shift-left: w414 -> [w426]
          shift-right: [w424] -> w413
          shift-left: w414 -> [w425]
          n192 = stacked-sequence {
            tunnel: w429 -> [w433 w438]
            tunnel: w428 -> [w430 _]
            tunnel: [_ w437] -> w427
            tunnel: w426 -> [_ w436]
            tunnel: w425 -> [_ w435]
            tunnel: [_ w434] -> w424
            frame #0 {
              n193 = call "3D_Traverse_move.vi"("Mode"=Trav_mode."Read traverse position", "Work in Tunnel Coordinates"=w430, "Simulate/Run"=User_Specific_mode."Run VI", "Traverse name"=w433) -> ()  [unwired: 5 in, 7 out]
            }
            frame #1 {
              n194 = global read "DriveConfigGlobal.vi" "Configurations"() -> (w439:T21[])
              n195 = for {
                tunnel: w439 -> [w449] mode=indexing
                tunnel: w438 -> [w446]
                shift-right: [w444] -> w437
                shift-left: w436 -> [w445]
                shift-right: [w440] -> w434
                shift-left: w435 -> [w441]
                i -> [w448]
                n196 = Unbundle By Name(w449) -> ("Channel Properties.Metadata Ch Name"=w443:string)
                n197 = Format Into String(format string="%d", initial string=w446, w448) -> (resulting string=w442:string)  [unwired: 1 in, 1 out]
                n198 = Build Array (concatenate)(w445, w443) -> (w444:string[])
                n199 = Build Array (concatenate)(w441, w442) -> (w440:string[])
              }
            }
          }
        }
        n200 = global write "Trav_pos_global.vi" "ADAM Positions Ch names"(w412) -> ()
        n201 = global write "Route_mapping_global.vi" "Display Mode"("Display Mode") -> ()
        n202 = global write "Trav_pos_global.vi" "Route checking Chs"(w413) -> ()
      }
      frame "Initialise Measurement Prog" {
        n203 = for {
          tunnel: w472 -> [w476] mode=indexing
          tunnel: [w475] -> w466 mode=indexing
          n204 = Unbundle By Name(w476) -> ("Meas Setup File"=w475:string)
        }
        n205 = call "Analyse_string_array.vi"("String array"=w466) -> ("Unique strings"=w465:string[])  [unwired: 1 in, 1 out]
        n206 = call "Perform_Meas_Setup.vi"("Simulate/Run"=User_Specific_mode."Check VI only", "String array"=w465) -> ("Continue?"=w467:bool)  [unwired: 1 out]
        n207 = Select(t=w470, s=w467, f=Multi_Run_Case."End" ("Multi Run Case")) -> (s? t:f=w469:T3)
      }
      frame "Input Current Position" {
        n208 = call "Save_ADAM_Table_Locally.vi"() -> ()  [unwired: 12 in]
      }
      frame "Experimental setup control" {
        n209 = global read "Trav_pos_global.vi" "Source Control?"() -> (w484:bool)
        n210 = Equal?(x=w487, y=User_Specific_mode."Run VI" ("Simulate/Run")) -> (x = y?=w486:bool)
        n211 = Or(x=w484, y=w486) -> (x .or. y?=w485:bool)
        n212 = case shown="True" w485 {
          tunnel: w484 -> [_ w491]
          frame False {
          }
          frame True {
            n213 = call "Exp_Setup_Control_remote.vi"("Dispersion?"=w491) -> ()  [unwired: 3 out]
          }
        }
        n214 = global write "Trav_pos_global.vi" "FFID Background"(T6 {"Start X"=nan, "Start Y"=nan, "Start Z"=nan, "End X"=nan, "End Y"=nan, "End Z"=nan, "No. of pts."=0, "Spacing"=enum."Linear", "Filename"=path "", "Tunnel Speed"=nan, "Averaging time (min)"=nan, "Extra Commands"="", "Specific Arguments"="", "Emission Rate (l/min)"=nan, "Trace Gas Concentration (%)"=nan, "Density Ratio"="", "Comments"="", "Row No"=0, "Row Type Selector"=enum."Blank Row", "Completion time"="", "Row Duration (mins)"=nan, "No. of Valid pts."=0, "Meas Setup File"=""} ("FFID Background")) -> ()
      }
      frame "Check source flowrates" {
        n215 = case shown="\"Run VI\"" w492 {
          tunnel: w493 -> [_ w502]
          frame "Check VI only", Default {
            n216 = Get Date/Time In Seconds() -> (seconds since 1Jan1904=w501:timestamp)
            n217 = global write "Trav_pos_global.vi" "Simulation Time"(w501) -> ()
          }
          frame "Run VI" {
            n218 = for {
              tunnel: w502 -> [w503] mode=indexing
              n219 = call "Set_Source.vi"("Source Status"=Client_Source_Status."Using", "Traverse line"=w503, "Simulate/Run"=User_Specific_mode."Check VI only") -> ()  [unwired: 1 in, 6 out]
            }
          }
        }
        n220 = Equal?(x=w492, y=User_Specific_mode."Run VI" ("Simulate/Run")) -> (x = y?=w496:bool)
        n221 = Increment(x=w498) -> (x+1=w494:T3)
        n222 = Select(t=w498, s=w496, f=w494) -> (s? t:f=w495:T3)
      }
      frame "Setup for running mode" {
        n223 = stacked-sequence {
          seq-local: [_ _ _ _ w539 _] -> [_ _ _ _ _ w557]
          tunnel: w509 -> [w514 _ _ w538 _ _]
          tunnel: w508 -> [_ _ w533 _ _ _]
          tunnel: [_ _ _ w536 _ _] -> w507
          tunnel: [_ _ _ _ w539 _] -> w506
          frame #0 {
            n224 = for {
              tunnel: w514 -> [w518] mode=indexing
              tunnel: [w515] -> w513 mode=indexing
              n225 = Unbundle By Name(w518) -> ("Row Type Selector"=w517:T8)
              n226 = Equal?(x=Multi_run_mode."Synchronize With:" ("Row Type Selector"), y=w517) -> (x = y?=w515:bool)
            }
            n227 = call "Setup_Environment.vi"() -> ()  [unwired: 1 in, 1 out]
            n228 = Or Array Elements(Boolean array=w513) -> (logical OR=w512:bool)
            n229 = case shown="True" w512 {
              frame False {
              }
              frame True {
                n230 = call "Declare_Sync_Client.vi"() -> ()  [unwired: 6 out]
              }
            }
          }
          frame #1 {
            n231 = Open VI Reference(vi path="Display_Trav_Views.vi" ("VI path")) -> (vi reference=w524:refnum<vi>, error out=w523:errorcluster)  [unwired: 1 in, 4 out]
            n232 = global write "Meas_global.vi" "Post Process"(Post_Process."Take New Data" ("Post Process")) -> ()
            n233 = property class="VI"(reference=w524, error in=w523, "Front Panel Window:Open"=FALSE) -> (reference out=w521:refnum<vi>, error out=w520:errorcluster)
            n234 = Close Reference(reference=w521, error in (no error)=w520) -> ()  [unwired: 1 out]
          }
          frame #2 {
            w528 = TRUE  # Start of Multi Run Prog
            w534 = TRUE
            n235 = Get Date/Time In Seconds() -> (seconds since 1Jan1904=w527:timestamp)
            n236 = To Double Precision Float(number=w527) -> (double precision float=w526:dbl)
            n237 = global write "Preference_global.vi" "Unblock Email"(w534) -> ()
            n238 = global write "Preference_global.vi" "Unblock SMS"(w534) -> ()
            n239 = global write "Meas_global.vi" "Start Time of experiment"(w526) -> ()
            n240 = local read "Command filename"() -> (w532:path)
            n241 = Path To String(path=w532) -> (string=w530:string)
            n242 = Concatenate Strings("Commencing a new multi run Prog having the setup filename of :" ("Message"), w530) -> (w529:string)
            n243 = call "Log_Current_row_to_Execute.vi"("Simulate/Run"=w533, "Message"=w529, "Start of Multi Run Prog"=w528) -> ()  [unwired: 2 in, 5 out]
          }
          frame #3 {
            n244 = call "Calc_Remaining_Time.vi"("Currently on Row"=-1, "Table In"=w538) -> ("Estimated Completion time"=w535:string, "Table Out"=w536:T6[])
            n245 = local write "Estimated Completion time"(w535) -> ()
            n246 = global write "Trav_pos_global.vi" "Estimated Completion time"(w535) -> ()
          }
          frame #4 {
            n247 = global read "Trav_pos_global.vi" "Source Control?"() -> (w540:bool)
            n248 = case shown="True" w540 {
              tunnel: [TRUE ("T button?") w545] -> w539
              frame False {
              }
              frame True {
                w546 = "EnFlo_Tunnel:Gas Solenoid:Status"
                n249 = Build Array(w546) -> (w549:string[])
                n250 = call "Get_Current_Scan_client.vi"("ADAM Ch Names"=w549) -> ("Numerical Values"=w548:dbl[])  [unwired: 3 out]
                n251 = Index Array(array=w548, index=0) -> (element=w544:dbl)
                n252 = Greater?(x=w544, y=0.5) -> (0:w542:bool)
                n253 = case shown="False" w542 {
                  tunnel: w546 -> [w555 _]
                  tunnel: [w550 TRUE ("T button?")] -> w545
                  frame False {
                    n254 = Format Into String(format string="The \"%s\" ADAM channel is showing that the blue gas button is not on.", w555) -> (resulting string=w553:string)  [unwired: 2 in, 1 out]
                    n255 = Two Button Dialog(message=w553, 1:"Stop" ("F button name (\"Cancel\")"), 2:"Continue" ("T button name (\"OK\")")) -> (T button?=w550:bool)
                  }
                  frame True {
                  }
                }
              }
            }
          }
          frame #5 {
            n256 = case shown="True" w557 {
              frame False {
              }
              frame True {
                n257 = call "Program_Active_Client.vi"("Mode"=enum16{"Program Active", "Traverse Level State"}."Traverse Level State", "Traverse level State"=Traverse_Level_State."Running") -> ()  [unwired: 1 in, 3 out]
              }
            }
          }
        }
      }
      frame "Skip Blank Rows" {
        n258 = stacked-sequence {
          tunnel: w564 -> [w567 w586]
          tunnel: w561 -> [w565 w582]
          frame #0 {
            n259 = Decrement(x=w567) -> (x-1=w566:i32)
            n260 = while {
              tunnel: w565 -> [w577]
              tunnel: w566 -> [w571]
              stop <- w568 continue-if-true
              n261 = local read "Currently on Row"() -> (w573:i32)
              n262 = Increment(x=w573) -> (x+1=w572:i32)
              n263 = Less?(x=w572, y=w571) -> (x < y?=w570:bool)
              n264 = Index Array(array=w577, index=w572) -> (element=w576:T6)
              n265 = Unbundle By Name(w576) -> ("Row Type Selector"=w575:T8)
              n266 = Equal?(x=Multi_run_mode."Blank Row" ("Row Type Selector"), y=w575) -> (x = y?=w569:bool)
              n267 = case shown="True" w569 {
                tunnel: w572 -> [_ w578]
                frame False {
                }
                frame True {
                  n268 = local write "Currently on Row"(w578) -> ()
                }
              }
              n269 = And(x=w569, y=w570) -> (x .and. y?=w568:bool)
            }
          }
          frame #1 {
            n270 = local read "Currently on Row"() -> (w584:i32)
            n271 = Increment(x=w584) -> (x+1=w583:i32)
            n272 = Index Array(array=w582, index=w583) -> (element=w585:T6)
            n273 = Unbundle By Name(w585) -> ("Row Type Selector"=w581:T8)
            n274 = Equal?(x=Multi_run_mode."Turn Off Row Repeating" ("Row Type Selector"), y=w581) -> (x = y?=w579:bool)
            n275 = while {
              shift-right: [w595] -> _
              shift-left: _ -> [w594]
              tunnel: w586 -> [w591]
              tunnel: w584 -> [w595]
              tunnel: w579 -> [w588]
              stop <- TRUE stop-if-true
              n276 = Decrement(x=w591) -> (x-1=w596:i32)
              n277 = Equal?(x=w595, y=w596) -> (x = y?=w589:bool)
              n278 = Not Equal?(x=w595, y=w594) -> (x != y?=w593:bool)
              n279 = Or(x=w588, y=w589) -> (x .or. y?=w587:bool)
              n280 = And(x=w593, y=w587) -> (x .and. y?=w592:bool)
              n281 = case shown="True" w592 {
                tunnel: w591 -> [_ w597]
                frame False {
                }
                frame True {
                  n282 = Initialize Array(timestamp(0 s since 1904-01-01) ("seconds since 1Jan1904"), w597) -> (w599:timestamp[])
                  n283 = global write "Trav_pos_global.vi" "Row completion times"(w599) -> ()
                }
              }
            }
          }
        }
      }
      frame "Which row to execute next" {
        # "Rep?"
        # "Repeat\nRow"
        n284 = local read "Currently on Row"() -> (w600:i32)
        n285 = stacked-sequence {
          seq-local: [_ w639 _] -> [_ _ w675]
          seq-local: [_ w638 _] -> [_ _ w676]
          seq-local: [w609 _ _] -> [_ w637 _]
          seq-local: [_ w634 _] -> [_ _ w669]
          tunnel: [w614 _ _] -> w606
          tunnel: w605 -> [w614 w641 w683]
          tunnel: w604 -> [_ _ w681]
          tunnel: w603 -> [_ w636 w682]
          tunnel: [_ _ w678] -> w602
          tunnel: w601 -> [_ _ w677]
          tunnel: w600 -> [w611 w633 w668]
          frame #0 {
            n286 = Array Size(array=w614) -> (size(s)=w613:i32)
            n287 = Decrement(x=w613) -> (x-1=w612:i32)
            n288 = Increment(x=w611) -> (x+1=w610:i32)
            n289 = while {
              tunnel: w610 -> [w618]
              tunnel: w614 -> [w630] mode=indexing
              tunnel: Multi_run_mode."Turn Off Row Repeating" ("Row Type Selector") -> [w629]
              tunnel: w612 -> [w625]
              tunnel: [w620] -> w609
              i -> [w622]
              stop <- w628 continue-if-true
              n290 = Less?(x=w622, y=w618) -> (x < y?=w623:bool)
              n291 = Unbundle By Name(w630) -> ("Row Type Selector"=w627:T8)
              n292 = Less?(x=w622, y=w625) -> (x < y?=w624:bool)
              n293 = Equal?(x=w622, y=w618) -> (x = y?=w619:bool)
              n294 = Equal?(x=w629, y=w627) -> (x = y?=w621:bool)
              n295 = case shown="True" w621 {
                tunnel: [TRUE w632] -> w620
                tunnel: w619 -> [_ w632]
                frame False {
                }
                frame True {
                }
              }
              n296 = Not(x=w621) -> (.not. x?=w626:bool)
              n297 = Compound Arithmetic op=AND(w626, w623, w624) -> (w628:bool)
            }
            n298 = global write "Trav_pos_global.vi" "Currently on point"(0 ("Currently on point")) -> ()
            n299 = global write "Trav_pos_global.vi" "Paused During Row?"(FALSE ("Paused During Row?")) -> ()
            n300 = global write "Trav_pos_global.vi" "Repeat Rows?"(w609) -> ()
          }
          frame #1 {
            n301 = global read "Trav_pos_global.vi" "Row completion times"() -> (w640:timestamp[])
            n302 = global read "Extra_Commands_Global.vi" "Minutes Before Repeating Row"() -> (w635:string)
            n303 = case shown="\"Run VI\"" w636 {
              tunnel: [w642 w643] -> w634
              frame "Check VI only" {
                n304 = global read "Trav_pos_global.vi" "Simulation Time"() -> (w642:timestamp)
              }
              frame "Run VI" {
                n305 = Get Date/Time In Seconds() -> (seconds since 1Jan1904=w643:timestamp)
                n306 = global write "Trav_pos_global.vi" "Simulation Time"(w643) -> ()
              }
            }
            n307 = while {
              tunnel: w641 -> [w653] mode=indexing
              tunnel: w640 -> [w656]
              tunnel: w634 -> [w655]
              tunnel: [w646] -> w639
              tunnel: [w645] -> w638
              tunnel: w637 -> [w649]
              tunnel: w633 -> [w647]
              tunnel: w635 -> [w644]
              i -> [w645]
              stop <- w652 continue-if-true
              n308 = Unbundle By Name(w653) -> ("Extra Commands"=w657:string)
              n309 = call "Extra_Commands.vi"("String to Search"=w657, "Command"=w644) -> ("Numeric Value"=w654:dbl, "Command Found"=w650:bool)  [unwired: 1 in, 3 out]
              n310 = And(x=w649, y=w650) -> (x .and. y?=w648:bool)
              n311 = case shown="True" w648 {
                tunnel: w656 -> [_ w663]
                tunnel: w655 -> [_ w664]
                tunnel: w645 -> [_ w662]
                tunnel: w654 -> [_ w660]
                tunnel: [FALSE w659] -> w646
                frame False {
                }
                frame True {
                  n312 = Index Array(array=w663, index=w662) -> (element=w665:timestamp)
                  n313 = Subtract(x=w664, y=w665) -> (x-y=w666:dbl)
                  n314 = Divide(x=w666, y=60.0) -> (x/y=w661:dbl)
                  n315 = Greater?(x=w661, y=w660) -> (0:w659:bool)
                }
              }
              n316 = Less?(x=w645, y=w647) -> (x < y?=w651:bool)
              n317 = Compound Arithmetic op=AND(invert w646, w651) -> (w652:bool)
            }
          }
          frame #2 {
            n318 = Not Equal?(x=w668, y=w676) -> (x != y?=w674:bool)
            n319 = And(x=w675, y=w674) -> (x .and. y?=w673:bool)
            n320 = case shown="False" w673 {
              tunnel: w676 -> [_ w709]
              tunnel: w668 -> [w705 w711]
              tunnel: [w704 w710] -> w679
              tunnel: [w704 w709] -> w670
              tunnel: w681 -> [w707 _]
              tunnel: [w703 TRUE] -> w680
              frame False {
                n321 = Increment(x=w705) -> (x+1=w706:i32)
                n322 = Greater?(x=w707, y=w706) -> (0:w703:bool)
                n323 = Select(t=w706, s=w703, f=w705) -> (s? t:f=w704:i32)
              }
              frame True {
                n324 = Greater?(x=w711, y=w709) -> (0:w712:bool)
                n325 = Select(t=w711, s=w712, f=w709) -> (s? t:f=w710:i32)
              }
            }
            n326 = global read "Trav_pos_global.vi" "Row completion times"() -> (w672:timestamp[])
            n327 = case shown="True" w680 {
              tunnel: w670 -> [_ w691]
              tunnel: w683 -> [_ w697]
              tunnel: w682 -> [w685 w689]
              tunnel: w679 -> [_ w695]
              tunnel: [w684 w694] -> w678
              tunnel: w677 -> [_ w694]
              frame False {
                n328 = case shown="\"Run VI\"" w685 {
                  tunnel: [Multi_Run_Case."Show jumped positions" ("Multi Run Case") Multi_Run_Case."Shut down source etc" ("Multi Run Case")] -> w684
                  frame "Check VI only" {
                  }
                  frame "Run VI" {
                  }
                }
              }
              frame True {
                n329 = Index Array(array=w697, index=w691) -> (element=w693:T6)
                n330 = Bundle By Name(cluster=w693, "Row No"=w691) -> (w692:T6)
                n331 = global write "Trav_pos_global.vi" "Meas Setup Number"(0 ("Meas Setup Number")) -> ()
                n332 = Build Array(w695) -> (w696:i32[])
                n333 = case shown="\"Run VI\"" w689 {
                  tunnel: w689 -> [_ w701]
                  tunnel: w692 -> [w698 w700]
                  tunnel: [w698 w699] -> w688
                  frame "Check VI only" {
                  }
                  frame "Run VI" {
                    n334 = call "Log_Current_row_to_Execute.vi"("Simulate/Run"=w701, "Start of Multi Run Prog"=FALSE, "Traverse line in"=w700) -> ("Traverse line Out"=w699:T6)  [unwired: 2 in, 4 out]
                  }
                }
                n335 = property on="Table" class="Arr (strict)"("Index Values"=w696) -> ()  [unwired: 2 in, 2 out]
                n336 = global write "Trav_pos_global.vi" "Current Row"(w688) -> ()
                "Currently on Row" <- w695
              }
            }
            n337 = Replace Array Subset(array=w672, new element=w669, index=w670) -> (w671:timestamp[])
            n338 = global write "Trav_pos_global.vi" "Row completion times"(w671) -> ()
          }
        }
      }
      frame "Evaluate IF Statement" {
        n339 = global read "Trav_pos_global.vi" "Current Row"() -> (w717:T6)
        n340 = Unbundle By Name(w717) -> ("Extra Commands"=w720:string)
        n341 = global read "Extra_Commands_Global.vi" "If Command"() -> (w723:string)
        n342 = call "Extra_Commands.vi"("String to Search"=w720, "Command"=w723) -> ("String Value"=w722:string, "Command Found"=w714:bool)  [unwired: 1 in, 3 out]
        n343 = Equal?(x=w718, y=User_Specific_mode."Run VI" ("Simulate/Run")) -> (x = y?=w713:bool)
        n344 = And(x=w714, y=w713) -> (x .and. y?=w715:bool)
        n345 = case shown="True" w715 {
          tunnel: w722 -> [_ w733]
          tunnel: [w729 w732] -> w716
          frame False {
            w729 = TRUE  # Execute Row?
          }
          frame True {
            n346 = call "Get_array_values_fr_String.vi"("String Value"=w733) -> ("Numeric Array"=w731:dbl[], "String array"=w730:string[])
            n347 = Index Array(array=w730, index=0 ("Index")) -> (element=w734:string)
            n348 = case shown="\"Global Value Between\"" w734 {
              tunnel: w733 -> [w739 _ _ _]
              tunnel: [w738 w740 w750 TRUE ("Execute Row?")] -> w732
              tunnel: w731 -> [_ w746 w764 _]
              tunnel: w730 -> [_ _ w758 _]
              frame "Time Between" {
                n349 = Get Date/Time In Seconds() -> (seconds since 1Jan1904=w736:timestamp)
                n350 = To Double Precision Float(number=w736) -> (double precision float=w737:dbl)
                n351 = call "If_Time_arguments.vi"("seconds since 1Jan1904"=w737, "String Value"=w739) -> ("Execute Row?"=w738:bool)  [unwired: 2 out]
              }
              frame "Global Value Between" {
                n352 = global read "Extra_Commands_Global.vi" "If command global value"() -> (w741:dbl)
                n353 = Index Array(array=w746, index=1 ("Index")) -> (element=w744:dbl)
                n354 = Index Array(array=w746, index=2 ("Index")) -> (element=w745:dbl)
                n355 = Max & Min(x=w744, y=w745) -> (max(x,y)=w743:dbl, min(x,y)=w742:dbl)
                n356 = In Range and Coerce(upper limit=w743, x=w741, lower limit=w742) -> (In Range?=w740:bool)  [unwired: 1 out]
              }
              frame "ADAM Channel Between" {
                n357 = Index Array(array=w758, index=1 ("Index")) -> (element=w757:string)
                n358 = Build Array(w757) -> (w756:string[])
                n359 = Index Array(array=w764, index=2 ("Index")) -> (element=w762:dbl)
                n360 = Index Array(array=w764, index=3 ("Index")) -> (element=w763:dbl)
                n361 = Max & Min(x=w762, y=w763) -> (max(x,y)=w761:dbl, min(x,y)=w760:dbl)
                n362 = call "Get_Current_Scan_client.vi"("ADAM Ch Names"=w756) -> ("Numerical Values"=w754:dbl[])  [unwired: 3 out]
                n363 = Index Array(array=w754, index=0 ("Index")) -> (element=w753:dbl)
                n364 = In Range and Coerce(upper limit=w761, x=w753, lower limit=w760) -> (In Range?=w751:bool)  [unwired: 1 out]
                n365 = Not A Number/Path/Refnum?(number/path/refnum=w753) -> (NaN/Path/Refnum?=w752:bool)
                n366 = Select(t=TRUE, s=w752, f=w751) -> (s? t:f=w750:bool)
              }
              frame "No Match", Default {
              }
            }
          }
        }
        n367 = Select(t=w726, s=w716, f=Multi_Run_Case."Calculate Row TIme" ("Multi Run Case")) -> (s? t:f=w725:T3)
      }
      frame "Perform Measurement Setup" {
        n368 = global read "Trav_pos_global.vi" "Current Row"() -> (w770:T6)
        n369 = case shown="\"Run VI\"" w769 {
          tunnel: w770 -> [_ w775]
          tunnel: w769 -> [_ w774]
          frame "Check VI only" {
          }
          frame "Run VI" {
            n370 = stacked-sequence {
              tunnel: w775 -> [w778 _]
              tunnel: w774 -> [w776 _]
              frame #0 {
                n371 = Unbundle By Name(w778) -> ("Extra Commands"=w777:string)
                n372 = call "Pause_for_server_ch_val.vi"("Extra command string"=w777, "Simulate/Run"=w776) -> ()  [unwired: 2 out]
              }
              frame #1 {
                n373 = Get Date/Time In Seconds() -> (seconds since 1Jan1904=w779:timestamp)
                n374 = To Double Precision Float(number=w779) -> (double precision float=w780:dbl)
                n375 = global write "Trav_pos_global.vi" "Start of Row time (Sec)"(w780) -> ()
              }
            }
          }
        }
      }
      frame "Set Measurement Conditions" {
        w786 = TRUE  # Row Completed
        w785 = FALSE  # Row Completed
        n376 = global read "Trav_pos_global.vi" "Current Row"() -> (w783:T6)
        n377 = Unbundle By Name(w783) -> ("Row Type Selector"=w788:T8)
        n378 = case shown="\"Run VI Named:\"" w788 {
          tunnel: [TRUE FALSE TRUE TRUE TRUE TRUE FALSE TRUE FALSE w837 FALSE FALSE FALSE] -> w793
          tunnel: w783 -> [w801 w804 w807 w810 w813 w816 w819 w822 w831 w836 w859 w862 w865]
          tunnel: [w801 w804 w807 w810 w813 w816 w819 w822 w830 w835 w859 w862 w865] -> w789
          tunnel: [w800 w803 w806 w809 w812 w815 w818 w821 w826 w833 w858 w861 w864] -> w787
          tunnel: w786 -> [w800 _ w806 w809 w812 _ _ _ _ w833 w858 w861 w864]
          tunnel: w785 -> [_ w803 _ _ _ w815 w818 w821 w826 _ _ _ _]
          tunnel: w782 -> [_ _ _ _ _ _ _ _ _ w834 _ _ _]
          frame "Move Traverse Only" {
          }
          frame "Check Beam Power" {
          }
          frame "Set Tunnel Speed Only" {
          }
          frame "Set Source Only" {
          }
          frame "Set Measurement Conditions" {
          }
          frame "Single Measurement" {
          }
          frame "Vertical Profile", Default {
          }
          frame "Scanning Valve Measurement" {
          }
          frame "Run VI Named:" {
            n379 = global read "Extra_Commands_Global.vi" "Skip Source Demand"() -> (w829:string)
            n380 = global read "Extra_Commands_Global.vi" "Establish Exp Conditions (s)"() -> (w825:string)
            n381 = Unbundle By Name(w831) -> ("Extra Commands"=w828:string)
            n382 = Concatenate Strings(w825, " = 0" ("Substring"), w829, w828) -> (w827:string)
            n383 = Bundle By Name(cluster=w831, "Extra Commands"=w827) -> (w830:T6)
          }
          frame "Send Message" {
            n384 = stacked-sequence {
              seq-local: [w838 _ _ _] -> [_ w843 _ _]
              tunnel: [_ _ _ FALSE] -> w837
              tunnel: w836 -> [_ w846 w852 w855]
              tunnel: [_ _ _ w855] -> w835
              tunnel: w834 -> [w839 _ _ _]
              frame #0 {
                n385 = Equal?(x=User_Specific_mode."Run VI" ("Simulate/Run"), y=w839) -> (x = y?=w838:bool)
              }
              frame #1 {
                n386 = Unbundle By Name(w846) -> ("Specific Arguments"=w844:string, "Filename"=w842:path)
                n387 = Build Array(w842) -> (w841:path[])
                n388 = case shown="True" w843 {
                  tunnel: "Message" ("Error Type") -> [_ w849]
                  tunnel: w844 -> [_ w848]
                  tunnel: w841 -> [_ w847]
                  frame False {
                  }
                  frame True {
                    n389 = call "Email_Text_Files.vi"("Filenames"=w847, "message"=w848, "subject ([No Subject])"=w849) -> ()
                  }
                }
              }
              frame #2 {
                n390 = global read "Extra_Commands_Global.vi" "Establish Exp Conditions (s)"() -> (w854:string)
                n391 = Unbundle By Name(w852) -> ("Extra Commands"=w853:string)
                n392 = call "Extra_Commands.vi"("String to Search"=w853, "Command"=w854) -> ("Numeric Value"=w850:dbl)  [unwired: 1 in, 4 out]
                n393 = call "Wait_Seconds_with_display.vi"("Message"="In Send Message Row", "Seconds to wait"=w850) -> ()  [unwired: 2 out]
              }
              frame #3 {
              }
            }
          }
          frame "Fall Back to this Row" {
          }
          frame "Turn Off Row Repeating" {
          }
          frame "Blank Row" {
          }
        }
        n394 = case shown="True" w793 {
          tunnel: w789 -> [_ w867]
          tunnel: w782 -> [_ w871]
          tunnel: [Multi_Run_Status."Continue" ("Status") w868] -> w781
          frame False {
          }
          frame True {
            w870 = 1  # Currently on Point
            n395 = call "Program_Active.vi"() -> ()  [unwired: 1 in]
            n396 = call "Set_Measurement_Conditions.vi"("Simulate/Run"=w871, "Currently on Point"=w870, "Traverse line"=w867) -> ("Status Cluster"=w869:T24)  [unwired: 2 out]
            n397 = Unbundle By Name(w869) -> ("Status"=w868:T2)
          }
        }
        n398 = case shown="\"Continue\"" w781 {
          tunnel: [w797 Multi_Run_Case."Calculate Row TIme" ("Multi Run Case")] -> w792
          tunnel: w791 -> [w798 _]
          tunnel: w787 -> [w795 _]
          frame "Continue" {
            n399 = Select(t=Multi_Run_Case."Calculate Row TIme" ("Multi Run Case"), s=w795, f=w798) -> (s? t:f=w797:T3)
          }
          frame "Jump to Next Point", Default {
          }
        }
        n400 = local write "Status"(w781) -> ()
      }
      frame "Execute Row" {
        n401 = global read "Trav_pos_global.vi" "Current Row"() -> (w873:T6)
        n402 = stacked-sequence {
          tunnel: w874 -> [w878 w889 w891]
          tunnel: w873 -> [w879 w886 w890]
          frame #0 {
            n403 = case shown="\"Check VI only\"" w878 {
              tunnel: w879 -> [w882 _]
              tunnel: w878 -> [w881 _]
              frame "Check VI only" {
                n404 = Unbundle By Name(w882) -> ("Extra Commands"=w883:string, "Row No"=w885:i32, "Meas Setup File"=w880:string)
                n405 = call "Skip_If Sd_Error_Below.vi"("String to Search"=w883, "Simulate/Run"=w881, "Measurement setup Applied?"=TRUE, "Row Number"=w885, "Measurement Setup File"=w880) -> ()  [unwired: 5 out]
              }
              frame "Run VI" {
              }
            }
          }
          frame #1 {
            n406 = call "Execute_Row.vi"("Simulate/Run"=w889, "Traverse line"=w886) -> ("Status"=w888:T2, "Traverse line out"=w887:T6)  [unwired: 2 out]
            n407 = global write "Trav_pos_global.vi" "Current Row"(w887) -> ()
            n408 = local write "Status"(w888) -> ()
          }
          frame #2 {
            w894 = FALSE  # Empty list
            n409 = call "Remember_RD_Folders.vi"("Empty list"=w894) -> ("List of Folders"=w893:path[])  [unwired: 1 in]
            n410 = for {
              tunnel: w890 -> [w899]
              tunnel: w893 -> [w898] mode=indexing
              tunnel: "Muti_Run_Log.xls" ("name or relative path") -> [w896]
              tunnel: w891 -> [w895]
              n411 = Build Path(base path=w898, name or relative path=w896) -> (appended path=w897:path)
              n412 = call "Log_Current_row_to_Execute.vi"("Simulate/Run"=w895, "Start of Multi Run Prog"=FALSE, "Traverse line in"=w899, "Multi Run Log File"=w897) -> ()  [unwired: 1 in, 5 out]
            }
          }
        }
      }
      frame "Calculate Row TIme" {
        n413 = global read "Trav_pos_global.vi" "Paused During Row?"() -> (w904:bool)
        n414 = local read "Status"() -> (w907:T2)
        n415 = global read "Trav_pos_global.vi" "Current Row"() -> (w903:T6)
        n416 = Equal?(x=w907, y=Multi_Run_Status."Continue" ("Status")) -> (x = y?=w906:bool)
        n417 = Equal?(x=w909, y=User_Specific_mode."Run VI" ("Simulate/Run")) -> (x = y?=w905:bool)
        n418 = Compound Arithmetic op=AND(w906, w905, invert w904) -> (w902:bool)
        n419 = case shown="False" w902 {
          tunnel: w903 -> [w922 w933]
          frame False {
            n420 = global read "Trav_pos_global.vi" "Simulation Time"() -> (w923:timestamp)
            n421 = To Double Precision Float(number=w923) -> (double precision float=w917:dbl)
            n422 = call "Calculate_Row_Time.vi"("Row Start Time (Sec Since 1904)"=w917, "Multi Run Row"=w922) -> ("Scalable Time (Sec)"=w920:dbl, "Fixed Time (Sec)"=w918:dbl)
            n423 = call "Overhead_Factor.vi"("Mode"=Overhead."Read Current Overhead") -> ("Current Overhead Factor"=w921:dbl)  [unwired: 3 in]
            n424 = Multiply(x=w921, y=w920) -> (x*y=w919:dbl)
            n425 = Add(x=w918, y=w919) -> (x+y=w914:dbl)
            n426 = global write "Trav_pos_global.vi" "Start of Row time (Sec)"(w914) -> ()
            n427 = Add(x=w917, y=w914) -> (x+y=w916:dbl)
            n428 = To Time Stamp(1:w916) -> (0:w915:timestamp)
            n429 = global write "Trav_pos_global.vi" "Simulation Time"(w915) -> ()
          }
          frame True {
            n430 = global read "Trav_pos_global.vi" "Start of Row time (Sec)"() -> (w931:dbl)
            n431 = Get Date/Time In Seconds() -> (seconds since 1Jan1904=w926:timestamp)
            n432 = To Double Precision Float(number=w926) -> (double precision float=w925:dbl)
            n433 = call "Calculate_Row_Time.vi"("Row Start Time (Sec Since 1904)"=w931, "Multi Run Row"=w933) -> ("Scalable Time (Sec)"=w927:dbl, "Fixed Time (Sec)"=w929:dbl)
            n434 = Subtract(x=w925, y=w931) -> (x-y=w930:dbl)
            n435 = Subtract(x=w930, y=w929) -> (x-y=w928:dbl)
            n436 = call "Overhead_Factor.vi"("Sum of Ideal times (Sec)"=w927, "Sum of Actual times (Sec)"=w928, "Mode"=Overhead."Update total times") -> ()  [unwired: 1 in, 1 out]
          }
        }
      }
      frame "Update time estimate" {
        n437 = global read "Trav_pos_global.vi" "Current Row"() -> (w937:T6)
        n438 = Unbundle By Name(w937) -> ("Row No"=w935:i32)
        n439 = local read "Currently on Row"() -> (w936:i32)
        n440 = Equal?(x=w935, y=w936) -> (x = y?=w934:bool)
        n441 = case shown="\"Run VI\"" w940 {
          tunnel: w943 -> [w951 w972]
          tunnel: [w950 w968] -> w942
          tunnel: w939 -> [_ w974]
          tunnel: [w949 w973] -> w938
          tunnel: w936 -> [w947 w967]
          tunnel: w937 -> [w948 w971]
          tunnel: w934 -> [w946 w970]
          frame "Check VI only" {
            n442 = global read "Trav_pos_global.vi" "Simulation Time"() -> (w953:timestamp)
            n443 = To Double Precision Float(number=w953) -> (double precision float=w952:dbl)
            n444 = call "Sec_to_date_filename.vi"("seconds"=w952) -> ("Day"=w955:string, "Time"=w954:string)  [unwired: 2 out]
            n445 = Concatenate Strings(w954, "  " ("Substring"), w955) -> (w949:string)
            n446 = case shown="True" w946 {
              tunnel: w947 -> [_ w966]
              tunnel: w951 -> [w957 w965]
              tunnel: [w957 w963] -> w950
              tunnel: w949 -> [_ w962]
              tunnel: w948 -> [_ w961]
              frame False {
              }
              frame True {
                n447 = global read "Trav_pos_global.vi" "Start of Row time (Sec)"() -> (w960:dbl)
                n448 = Divide(x=w960, y=60.0) -> (x/y=w958:dbl)
                n449 = Bundle By Name(cluster=w961, "Completion time"=w962, "Row Duration (mins)"=w958) -> (w964:T6)
                n450 = Replace Array Subset(array=w965, new element=w964, index=w966) -> (w963:T6[])
              }
            }
          }
          frame "Run VI" {
            n451 = case shown="True" w970 {
              tunnel: w967 -> [_ w981]
              tunnel: w972 -> [w977 w980]
              tunnel: w971 -> [_ w979]
              tunnel: [w977 w978] -> w969
              frame False {
              }
              frame True {
                n452 = Replace Array Subset(array=w980, new element=w979, index=w981) -> (w978:T6[])
              }
            }
            n453 = call "Calc_Remaining_Time.vi"("Currently on Row"=w967, "Table In"=w969) -> ("Table Out"=w968:T6[])  [unwired: 1 out]
            n454 = Decrement(x=w974) -> (x-1=w976:i32)
            n455 = Index Array(array=w968, index=w976) -> (element=w975:T6)
            n456 = Unbundle By Name(w975) -> ("Completion time"=w973:string)
          }
        }
        "Estimated Completion time" <- w938
        n457 = global write "Trav_pos_global.vi" "Estimated Completion time"(w938) -> ()
      }
      frame "Pause Multi Run Program" {
        n458 = while {
          tunnel: "Pause" -> [w993]
          tunnel: [w996] -> w988
          tunnel: w987 -> [w995]
          tunnel: w985 -> [w994]
          shift-right: [w993] -> _
          shift-left: _ -> [w992]
          stop <- TRUE stop-if-true
          n459 = case shown="True" w993 {
            tunnel: [w997 w1002] -> w996
            tunnel: w995 -> [w997 w1000]
            tunnel: w994 -> [_ w1001]
            tunnel: w993 -> [_ w999]
            tunnel: w992 -> [_ w998]
            frame False {
            }
            frame True {
              n460 = stacked-sequence {
                tunnel: w1000 -> [_ _ _ _ w1017]
                tunnel: [_ _ _ _ w1018] -> w1002
                tunnel: w1001 -> [w1004 _ _ _ _]
                tunnel: w999 -> [_ _ _ w1013 _]
                tunnel: w998 -> [_ _ _ w1012 _]
                frame #0 {
                  n461 = Quotient & Remainder(x=w1004, y=15) -> (x-y*floor(x/y)=w1003:i32)  [unwired: 1 out]
                  n462 = case shown="0" w1003 {
                    frame 0 {
                      n463 = Current VI's Path() -> (path=w1006:path)
                      n464 = call "Bring_to_front.vi"("path"=w1006) -> ()
                    }
                    frame 1, Default {
                    }
                  }
                }
                frame #1 {
                  n465 = global write "Trav_pos_global.vi" "Paused During Row?"(TRUE ("Paused During Row?")) -> ()
                  "Pause message" <- "Multi Run Program Paused!!!!" ("Pause message")
                }
                frame #2 {
                  n466 = property on="Pause message" class="Str"("Visible"=TRUE) -> ()  [unwired: 2 in, 2 out]
                  n467 = Wait Until Next ms Multiple(millisecond multiple=u32 1500) -> ()  [unwired: 1 out]
                }
                frame #3 {
                  n468 = Compound Arithmetic op=AND(w1013, invert w1012) -> (w1011:bool)
                  n469 = case shown="True" w1011 {
                    frame False {
                    }
                    frame True {
                      n470 = call "Program_Active_Client.vi"("Mode"=enum16{"Program Active", "Traverse Level State"}."Program Active", "Time till next contact (Sec)"=12000.0, "Traverse level State"=Traverse_Level_State."Running") -> ()  [unwired: 3 out]
                    }
                  }
                }
                frame #4 {
                  n471 = property on="Pause message" class="Str"("Visible"=FALSE) -> ()  [unwired: 2 in, 2 out]
                  n472 = Wait Until Next ms Multiple(millisecond multiple=u32 1500) -> ()  [unwired: 1 out]
                  n473 = Decrement(x=w1017) -> (x-1=w1018:T3)
                }
              }
            }
          }
        }
        n474 = call "Overhead_Factor.vi"("Mode"=Overhead."Read Current Overhead") -> ("Current Overhead Factor"=→"Current Overhead Factor":dbl)  [unwired: 3 in]
      }
      frame "Do Another Row?" {
        w1031 = Multi_Run_Status."Terminate Run" ("Status")
        n475 = case shown="False" "Stop after Repeats" {
          tunnel: [w1039 w1040] -> w1025
          tunnel: w1021 -> [_ w1041]
          frame False {
            n476 = local read "Currently on Row"() -> (w1039:i32)
            n477 = Increment(x=w1039) -> (x+1=→"Last Row Run":i32)
          }
          frame True {
            n478 = Decrement(x=w1041) -> (x-1=w1040:i32)
            n479 = local write "Currently on Row"(w1040) -> ()
          }
        }
        n480 = case shown="False" "stop" {
          tunnel: [w1042 w1043] -> w1032
          tunnel: w1031 -> [_ w1043]
          frame False {
            n481 = local read "Status"() -> (w1042:T2)
          }
          frame True {
            n482 = local write "Status"(w1043) -> ()
          }
        }
        n483 = Not Equal?(x=w1032, y=w1031) -> (x != y?=w1030:bool)
        n484 = Increment(x=w1025) -> (x+1=w1024:i32)
        n485 = Index Array(array=w1026, index=w1024) -> (element=w1023:T6)
        n486 = Unbundle By Name(w1023) -> ("Row Type Selector"=w1029:T8)
        n487 = Equal?(x=w1029, y=Multi_run_mode."Turn Off Row Repeating" ("Row Type Selector")) -> (x = y?=w1027:bool)
        n488 = case shown="True" w1030 {
          tunnel: [w1044 w1048] -> w1036
          tunnel: w1025 -> [_ _]
          tunnel: w1035 -> [w1045 _]
          tunnel: w1026 -> [_ _]
          tunnel: w1032 -> [_ w1049]
          tunnel: w1021 -> [_ _]
          tunnel: w1027 -> [_ _]
          frame False {
            n489 = case shown="\"Check VI only\"" w1045 {
              tunnel: [Multi_Run_Case."Show jumped positions" ("Multi Run Case") Multi_Run_Case."Shut down source etc" ("Multi Run Case")] -> w1044
              frame "Check VI only" {
              }
              frame "Run VI" {
              }
            }
          }
          frame True {
            n490 = case shown="\"Jump To Fall Back\"" w1049 {
              tunnel: [Multi_Run_Case."Skip Blank Rows" ("Multi Run Case") Multi_Run_Case."Find Next Fall Back Row" ("Multi Run Case")] -> w1048
              frame "Continue", Default {
              }
              frame "Jump To Fall Back" {
              }
            }
          }
        }
      }
      frame "Find Next Fall Back Row" {
        n491 = local read "Currently on Row"() -> (w1053:i32)
        n492 = Increment(x=w1053) -> (x+1=w1052:i32)
        n493 = Index Array(array=w1061, index=w1053) -> (element=w1062:T6)
        n494 = Array Size(array=w1061) -> (size(s)=w1060:i32)
        n495 = Unbundle By Name(w1062) -> ("Row Type Selector"=w1056:T8)
        n496 = Greater?(x=w1060, y=w1052) -> (0:w1059:bool)
        n497 = Equal?(x=w1056, y=Multi_run_mode."Fall Back to this Row" ("Mode")) -> (x = y?=w1054:bool)
        n498 = case shown="True" w1059 {
          tunnel: [Multi_Run_Case."Skip Blank Rows" ("Multi Run Case") w1069] -> w1058
          tunnel: w1054 -> [_ w1065]
          tunnel: w1053 -> [_ w1066]
          frame False {
          }
          frame True {
            n499 = case shown="False" w1065 {
              tunnel: w1066 -> [w1071 _]
              frame False {
                n500 = Increment(x=w1071) -> (x+1=w1070:i32)
                n501 = local write "Currently on Row"(w1070) -> ()
              }
              frame True {
              }
            }
            n502 = Select(t=Multi_Run_Case."Skip Blank Rows" ("Multi Run Case"), s=w1065, f=Multi_Run_Case."Find Next Fall Back Row" ("Multi Run Case")) -> (s? t:f=w1069:T3)
          }
        }
      }
      frame "Shut down source etc" {
        n503 = for {
          tunnel: w1091 -> [w1110] mode=indexing
          tunnel: Multi_run_mode."Synchronize With:" ("Mode") -> [w1108]
          tunnel: [w1107] -> w1093 mode=indexing
          n504 = Unbundle By Name(w1110) -> ("Row Type Selector"=w1109:T8)
          n505 = Equal?(x=w1109, y=w1108) -> (x = y?=w1107:bool)
        }
        n506 = call "Overhead_Factor.vi"("Mode"=Overhead."Re Scale totals to 3 hrs") -> ()  [unwired: 3 in, 1 out]
        n507 = local read "Status"() -> (w1079:T2)
        n508 = call "Set_Source.vi"("Source Status"=Client_Source_Status."Not Using", "Simulate/Run"=w1082) -> ("Status Cluster"=w1083:T24)  [unwired: 2 in, 5 out]
        n509 = call "Program_Active_Client.vi"("Mode"=enum16{"Program Active", "Traverse Level State"}."Traverse Level State", "Traverse level State"=Traverse_Level_State."Complete") -> ()  [unwired: 1 in, 3 out]
        n510 = global read "Meas_global.vi" "Start Time of experiment"() -> (w1089:dbl)
        n511 = Equal?(x=w1079, y=Multi_Run_Status."Terminate Run" ("Status")) -> (x = y?=w1077:bool)
        n512 = call "Prog_Status_Handler.vi"("Status Cluster"=w1083, "Simulate/Run"=w1082) -> ()  [unwired: 2 out]
        n513 = global read "Meas_global.vi" "LDA data"() -> (w1098:enum16{"No LDA data", "Take LDA data"})
        n514 = Or Array Elements(Boolean array=w1093) -> (logical OR=w1080:bool)
        n515 = Get Date/Time In Seconds() -> (seconds since 1Jan1904=w1072:timestamp)
        n516 = Compound Arithmetic op=AND(w1080, invert w1077) -> (w1081:bool)
        n517 = To Double Precision Float(number=w1072) -> (double precision float=w1090:dbl)
        n518 = case shown="\"Take LDA data\"" w1098 {
          frame "No LDA data" {
          }
          frame "Take LDA data" {
            w1111 = FALSE  # High Voltage
            w1116 = 0.0  # Input
            n519 = global read "LDA_meas_global_2.vi" "BSA2 info"() -> (w1113:T25)
            n520 = global read "LDA_meas_global_1.vi" "BSA1 info"() -> (w1115:T25)
            n521 = Unbundle By Name(w1113) -> ("GPIB Address"=w1112:string)
            n522 = Unbundle By Name(w1115) -> ("GPIB Address"=w1114:string)
            n523 = call "Hydrosonic_Conrol.vi"("Input Mode"=enum16{"Desired Frequency", "Transducer value"}."Transducer value", "Desired Value"=w1116) -> ()  [unwired: 2 in, 2 out]
            n524 = call "Set_BSA_voltage_On_Off.vi"("GPIB address"=w1114, "High Voltage"=w1111) -> ()  [unwired: 1 in, 5 out]
            n525 = call "Set_BSA_voltage_On_Off.vi"("GPIB address"=w1112, "High Voltage"=w1111) -> ()  [unwired: 1 in, 5 out]
          }
        }
        n526 = case shown="True" w1081 {
          frame False {
          }
          frame True {
            n527 = global read "Preference_global.vi" "Rig Setup"() -> (w1100:string)
            n528 = Concatenate Strings(w1100, ":Program:Sync") -> (w1102:string)
            n529 = Bundle By Name(cluster=T19 {"Channel Name"="", "New Value"=0.0} ("Update Scan Value Cluster"), "Channel Name"=w1102, "New Value"=1000.0 ("Bundle Element")) -> (w1103:T19)
            n530 = Build Array(w1103) -> (w1105:T19[])
            n531 = call "Update_Current_Value_client.vi"("Update array in"=w1105) -> ()  [unwired: 1 in]
          }
        }
        n532 = Subtract(x=w1090, y=w1089) -> (x-y=w1088:dbl)
        n533 = Greater?(x=w1088, y=300.0) -> (0:w1085:bool)
        n534 = Not(x=w1085) -> (.not. x?=→"Non Starter":bool)
        n535 = Increment(x=w1075) -> (x+1=w1074:T3)
        n536 = Increment(x=w1074) -> (x+1=w1073:T3)
        n537 = Select(t=w1075, s=w1085, f=w1073) -> (s? t:f=w1086:T3)
      }
      frame "Email results to users" {
        n538 = local read "Currently on Row"() -> (w1123:i32)
        n539 = Increment(x=w1123) -> (x+1=w1118:i32)
        n540 = Split 1D Array(array=w1120, index=w1118) -> (first subarray=w1127:T6[], second subarray=w1126:T6[])
        n541 = Array Size(array=w1126) -> (size(s)=w1128:i32)
        n542 = for {
          tunnel: w1127 -> [w1143] mode=indexing
          shift-right: [w1141] -> w1129
          shift-left: string[] [] -> [w1142]
          n543 = Unbundle By Name(w1143) -> ("Row Type Selector"=w1134:T8, "Filename"=w1140:path, "Comments"=w1139:string)
          n544 = Not Equal?(x=Multi_run_mode."Auto Calibrate" ("Row Type Selector"), y=w1134) -> (x != y?=w1136:bool)
          n545 = Empty String/Path?(string/path=w1140) -> (empty?=w1137:bool)
          n546 = Compound Arithmetic op=AND(w1136, invert w1137) -> (w1135:bool)
          n547 = case shown="True" w1135 {
            tunnel: w1142 -> [w1144 w1152]
            tunnel: [w1144 w1151] -> w1141
            tunnel: w1140 -> [_ w1150]
            tunnel: w1139 -> [_ w1148]
            frame False {
            }
            frame True {
              n548 = Path To String(path=w1150) -> (string=w1149:string)
              n549 = Match Pattern(string=w1148, regular expression=" !!Program added comments") -> (after substring=w1145:string)  [unwired: 4 out]
              n550 = Concatenate Strings(w1149, w1145) -> (w1147:string)
              n551 = Build Array (concatenate)(w1152, w1147) -> (w1151:string[])
            }
          }
        }
        n552 = Equal To 0?(x=w1128) -> (x = 0?=w1119:bool)
        n553 = case shown="False" w1119 {
          tunnel: ["Having completed only some of the requested rows." ("Message") ""] -> w1124
          frame False {
          }
          frame True {
          }
        }
        n554 = call "End_of_run_messages.vi"("Message"=w1124, "Subject"="Multi Run Ended", "Attachments"=w1129) -> ()  [unwired: 1 in]
      }
      frame "Save run efficiency" {
        w1164 = FALSE  # append to file? (new file:F)
        w1163 = FALSE  # advisory dialog? (display:T)
        n555 = call "Setup_Filepath.vi"("Setup File Type"=Setup_Filetype."General", "Filename in"="Preferences.xls" ("name or relative path")) -> ("Filename Out"=w1153:path)  [unwired: 1 out]
        n556 = call "Overhead_Factor.vi"("Mode"=Overhead."Read Current Overhead") -> ("Current Overhead Factor"=w1158:dbl)  [unwired: 3 in]
        n557 = Number To Fractional String(number=w1158, precision (6)=i16 4) -> (F-format string=w1156:string)  [unwired: 2 out]
        n558 = call "Read_Characters_From_File.ph.vi"("file path (dialog if empty)"=w1153) -> ("character string"=w1161:string)  [unwired: 1 in, 7 out]
        n559 = call "Replace_data_in_setup_string.vi"("New data string"=w1156, "Input string"=w1161, "Variable name"="Current Overhead Factor") -> ("Appended string"=w1160:string)
        n560 = call "Write_Characters_To_File.vi"("file path (dialog if empty)"=w1153, "advisory dialog? (display:T)"=w1163, "character string"=w1160, "append to file? (new file:F)"=w1164) -> ()  [unwired: 1 in, 4 out]
      }
      frame "Remove Skipped Commands" {
        n561 = for {
          tunnel: w1170 -> [w1178] mode=indexing
          tunnel: [w1177] -> w1169 mode=indexing
          n562 = Unbundle By Name(w1178) -> ("Comments"=w1176:string)
          n563 = Match Pattern(string=w1176, regular expression=" !!Program added comments") -> (before substring=w1175:string)  [unwired: 4 out]
          n564 = Bundle By Name(cluster=w1178, "Comments"=w1175) -> (w1177:T6)
        }
      }
      frame "Show jumped positions" {
        n565 = global read "Trav_pos_global.vi" "Jumped Positions"() -> (w1181:dbl[][])
        n566 = Array Size(array=w1181) -> (size(s)=w1184:i32[])
        n567 = Index Array(array=w1184, index=0) -> (element=w1180:i32)
        n568 = Greater Than 0?(x=w1180) -> (x > 0?=w1182:bool)
        n569 = case shown="True" w1182 {
          tunnel: w1181 -> [_ w1195]
          tunnel: w1180 -> [_ w1194]
          frame False {
            w1188 = TRUE  # Front Panel Window:Is Frontmost
            n570 = Current VI's Path() -> (path=w1189:path)
            n571 = Open VI Reference(vi path=w1189) -> (vi reference=w1190:refnum<vi>, error out=w1191:errorcluster)  [unwired: 1 in, 4 out]
            n572 = property class="VI"(reference=w1190, error in=w1191, "Front Panel Window:Is Frontmost"=w1188) -> (reference out=w1192:refnum<vi>, error out=w1193:errorcluster)
            n573 = Close Reference(reference=w1192, error in (no error)=w1193) -> ()  [unwired: 1 out]
          }
          frame True {
            n574 = stacked-sequence {
              tunnel: w1195 -> [w1196 w1206]
              tunnel: w1194 -> [w1200 _]
              frame #0 {
                n575 = global read "Trav_pos_global.vi" "Default Traverse Setup"() -> (w1197:string)
                n576 = Format Into String(format string="There are %d points which cannot be reached", w1200) -> (resulting string=w1198:string)  [unwired: 2 in, 1 out]
                n577 = call "Display_Trav_Views.vi"("Current Probe Position"=w1196, "Traverse Name"=w1197, "Open Front Panel"=TRUE, "Error Comments"=w1198, "Crash?"=FALSE) -> ()  [unwired: 2 in, 4 out]
              }
              frame #1 {
                n578 = local read "Command filename"() -> (w1210:path)
                n579 = Array To Spreadsheet String(array=w1206, 3:"%.1f" ("format string")) -> (spreadsheet string=w1204:string)  [unwired: 1 out]
                n580 = Strip Path(path=w1210) -> (stripped path=w1209:path)  [unwired: 1 out]
                n581 = Build Path(base path=w1209, name or relative path="Jumped_Positions.xls") -> (appended path=w1207:path)
                n582 = call "Write_File_Simple.vi"("append to file? (new file:F)"=FALSE, "character string"=w1204, "file path"=w1207) -> ()  [unwired: 2 out]
              }
            }
          }
        }
      }
      frame "Save Setup to File" {
        w1227 = FALSE  # Start of Multi Run Prog
        n583 = Array Size(array=w1241) -> (size(s)=w1246:i32)
        n584 = local read "Last Row Run"() -> (w1216:i32)
        n585 = local read "Status"() -> (w1222:T2)
        n586 = local read "Stop after Repeats"() -> (w1225:bool)
        n587 = local read "stop"() -> (w1226:bool)
        n588 = Decrement(x=w1216) -> (x-1=w1217:i32)
        n589 = Increment(x=w1217) -> (x+1=w1229:i32)
        n590 = local read "Command filename"() -> (w1212:path)
        n591 = Equal?(x=w1222, y=Multi_Run_Status."Continue" ("Status")) -> (x = y?=w1221:bool)
        n592 = Compound Arithmetic op=OR(w1225, w1226, w1221) -> (w1224:bool)
        n593 = local read "Non Starter"() -> (w1234:bool)
        n594 = Select(t=w1229, s=w1224, f=w1217) -> (s? t:f=w1228:i32)
        n595 = Less?(x=w1220, y=T9."Run Multi Run Prog") -> (x < y?=w1218:bool)
        n596 = Equal?(x=w1246, y=w1216) -> (x = y?=w1236:bool)
        n597 = Equal To 0?(x=w1229) -> (x = 0?=w1235:bool)
        n598 = Split 1D Array(array=w1241, index=w1228) -> (second subarray=w1244:T6[])  [unwired: 1 out]
        n599 = Compound Arithmetic op=OR(w1236, w1235, w1234, w1218) -> (w1237:bool)
        n600 = call "Current_Filepath.vi"("Filename in"=w1212, "Data Type"="Commands") -> ("Filename Out"=w1211:path)  [unwired: 1 out]
        n601 = local read "Work in Tunnel Coordinates?"() -> (w1215:T1)
        n602 = local read "Jump Bad Positions"() -> (w1214:bool)
        n603 = case shown="False" w1237 {
          tunnel: w1211 -> [w1254 w1287]
          tunnel: [w1253 w1287] -> w1245
          tunnel: w1244 -> [w1251 _]
          tunnel: [w1250 w1288] -> w1243
          tunnel: w1241 -> [w1252 w1288]
          tunnel: w1215 -> [w1249 _]
          tunnel: w1214 -> [w1248 _]
          frame False {
            n604 = stacked-sequence {
              tunnel: w1254 -> [w1255 w1266 _]
              tunnel: [_ w1259 _] -> w1253
              tunnel: w1252 -> [w1258 _ w1271]
              tunnel: w1251 -> [_ _ w1269]
              tunnel: [_ _ w1268] -> w1250
              tunnel: w1249 -> [w1257 _ _]
              tunnel: w1248 -> [w1256 _ _]
              frame #0 {
                n605 = call "Save_Trav_setup.vi"("Work in Tunnel Coordinates?"=w1257, "Trav Table"=w1258, "Jump Bad Positions"=w1256, "Setup filename"=w1255) -> ()  [unwired: 2 out]
              }
              frame #1 {
                n606 = Strip Path(path=w1266) -> (stripped path=w1267:path, name=w1265:string)
                n607 = call "Add_filename_suffix.vi"("Filename"=w1265) -> ("Original Suffix"=w1262:string, "Base name"=w1264:string)  [unwired: 1 in, 2 out]
                n608 = Concatenate Strings(w1264, "_Rem", w1262) -> (w1261:string)
                n609 = Build Path(base path=w1267, name or relative path=w1261) -> (appended path=w1260:path)
                n610 = call "Find_Unique_Filename.vi"("Path In"=w1260) -> ("Unique Path Out"=w1259:path)  [unwired: 1 in, 1 out]
              }
              frame #2 {
                n611 = Index Array(array=w1271, index=0) -> (element=w1274:T6)
                n612 = Initialize Array(w1274, 0 ("dimension size")) -> (w1273:T6[])
                n613 = global read "Extra_Commands_Global.vi" "Minutes Before Repeating Row"() -> (w1272:string)
                n614 = for {
                  shift-right: [w1277] -> w1270
                  shift-left: w1273 -> [w1279]
                  tunnel: w1272 -> [w1281]
                  tunnel: w1271 -> [w1278] mode=indexing
                  n615 = Unbundle By Name(w1278) -> ("Extra Commands"=w1280:string)
                  n616 = call "Extra_Commands.vi"("String to Search"=w1280, "Command"=w1281) -> ("Command Found"=w1282:bool)  [unwired: 1 in, 4 out]
                  n617 = case shown="False" w1282 {
                    tunnel: w1279 -> [w1283 w1286]
                    tunnel: w1278 -> [_ w1285]
                    tunnel: [w1283 w1284] -> w1277
                    frame False {
                    }
                    frame True {
                      n618 = Build Array (concatenate)(w1286, w1285) -> (w1284:T6[])
                    }
                  }
                }
                n619 = Build Array (concatenate)(w1270, w1269) -> (w1268:T6[])
              }
            }
          }
          frame True {
          }
        }
        n620 = Path To String(path=w1211) -> (string=w1233:string)
        n621 = Concatenate Strings("Multi run Prog Ended having the setup filename of :" ("Message"), w1233) -> (w1232:string)
        n622 = call "Save_Trav_setup.vi"("Work in Tunnel Coordinates?"=w1215, "Trav Table"=w1243, "Jump Bad Positions"=w1214, "Setup filename"=w1245) -> ("Trav Table Out"=w1242:T6[])  [unwired: 1 out]
        n623 = call "Log_Current_row_to_Execute.vi"("Simulate/Run"=w1231, "Message"=w1232, "Start of Multi Run Prog"=w1227) -> ()  [unwired: 2 in, 5 out]
        n624 = Select(t=w1242, s=w1237, f=w1241) -> (s? t:f=w1240:T6[])
      }
      frame "End" {
        w1290 = ""
        w1292 = path ""
        w1293 = 0 ("No. of pts.")
        w1295 = nan
        n625 = global write "Trav_pos_global.vi" "Top level setup filename"(w1292) -> ()
        n626 = global read "Trav_pos_global.vi" "Current Row"() -> (w1299:T6)
        n627 = Bundle By Name(cluster=w1299, "Start X"=w1295, "Start Y"=w1295, "Start Z"=w1295, "End X"=w1295, "End Y"=w1295, "End Z"=w1295, "No. of pts."=w1293, "Spacing"=Spacing."Linear", "Filename"=w1292, "Tunnel Speed"=w1295, "Averaging time (min)"=w1295, "Extra Commands"=w1290, "Specific Arguments"=w1290, "Emission Rate (l/min)"=w1295, "Trace Gas Concentration (%)"=w1295, "Density Ratio"=w1290, "Comments"=w1290, "Row No"=w1293, "Row Type Selector"=Multi_run_mode."Blank Row", "Completion time"=w1290, "Meas Setup File"=w1290, "Row Duration (mins)"=w1295, "No. of Valid pts."=w1293) -> (w1298:T6)
        n628 = Current VI's Path() -> (path=w1291:path)
        n629 = global write "Trav_pos_global.vi" "Current Row"(w1298) -> ()
        n630 = global write "Trav_pos_global.vi" "Meas Setup Number"(0 ("Meas Setup Number")) -> ()
        n631 = call "Bring_to_front.vi"("path"=w1291) -> ()
        n632 = global write "Trav_pos_global.vi" "Estimated Completion time"("") -> ()
        n633 = Build Array(u32 0) -> (w1300:u32[])
        n634 = property on="Table" class="Arr (strict)"("Index Values"=w1300) -> ()  [unwired: 2 in, 2 out]
      }
    }
    n635 = case shown="False" w8 {
      tunnel: w4 -> [_ w15]
      frame False {
      }
      frame True {
        n636 = local write "Table"(w15) -> ()
      }
    }
    "Multi Run Case" <- w10
  }
